vi "GUI_Beampointing2_TRA.vi"() -> ()   [LabVIEW 2013]
uses:
  shared programs/GUI_Template/GUI_master/tcp_new_data_event.ctl
  shared programs/GUI_Template/GUI_master/tcp new data cluster.ctl
  Device Driver/TRAServer/StatusTRA_TypDef.ctl
  Ctrs/beam detection.ctl
  Ctrs/move.ctl
  Ctrs/stats.ctl
  <vilib>/Analysis/NI_AALBase.lvlib
  Device Driver/TRAServer/TRAServer.lvclass
panel:
  in  "Status.Axis 1::2":T1=enum."DISABLE"
  in  "Status.Axis 2::2":T1=enum."DISABLE" caption="Status.Axis 1::2"
  in  "UDP error message":string
  in  "Set Centriod Target":bool
  in  "Tab Control 2":enum32{"CCD Original ", "CCD Detected"}(tab)=enum."CCD Detected"
  out "image::1":T2(plugin-control) caption="StagingM1Far"
  out "Beam":T2(plugin-control)
  in  "Reset History":bool
  out "centriod X":dbl[](graph)=[269.2727355957031, 269.2727355957031, 269.3190002441406]
  out "centriod Y":dbl[](graph)=[287.58294677734375, 287.58294677734375, 287.771484375]
  out "Stats":cluster{timestamp[], dbl[]}[](graph)
  out "move.Stepsize 2":dbl
  out "move.Stepsize":dbl
  in  "Tab Control":enum32{"System", "Detection", "Feedback"}(tab)=enum."Detection"
  in  "Save Stats":bool
  in  "update speed [ms]":i32=200
  in  "img to avg":i32=10
  in  "Save Config":bool
  in  "Load Config":bool
  in  "Cameras":u16(ring)=15 items=["Amp2_surfEast", "Amp2_surfWest", "amp3_surfeast", "amp3_surfwest", "BELLAFrontendCompCam", "Bella_LP_Mode", "Bella_TopviewCCD", "Comp_Final", "EBeam_Profile_BELLA_1", "Flea1_Lanex", "Flea3FW2x2_Lanex", "FLea3Gig_Lanex", "HeatHPDCCD", "HPD_CCD", "LB-FiberCam", "M1-Back-Cam", "M1Cam", "M2Cam", "M3HPD_CCD", "M3HPD_CCD_Near", "M4Cam", "M5Cam", "MagSpecA", "MagSpecB", "MagSpecC", "MagSpecD", "MagSpecE", "MagSpecF", "MagSpecG", "MagSpecH", "MagSpecI", "MagSpecJ", "MagSpecK", "MagSpecL", "P1-SideView", "P2-BlackGuppy", "P2-capspec", "P2-Guppy", "P2-HeatCamPost", "P2-HeatCamPostNear", "P2-HeatCamPreFar", "P2-HeatCamPreFarA", "P2-HeatCamPreNear", "P2-phasics", "P2-phasics151", "P2-ProbeCamPost", "P2-ProbeCamPostNear", "P2-ProbeCamPreNear", "P2-TempCam", "PL1-HexCam", "PL1-phasics151", "PL1-SideSpec", "PL1-TopSpc", "PriyankaCam", "SimCam", "TDBfarfield", "TDBnearfield", "Tel4_Cam", "TPL-Cam-Faraday"]
  in  "wait":u32=200
  in  "beam detection para":T3={"Filter"=1, "Filter Para"={"X Size"=5, "Y Size"=5, "% Tolerance"=1}, "detection method"=4, "smal para"=[{"Measurement Parameter"=35, "Range Lower Value"=0.0, "Range Upper Value"=500.0, "Range"=TRUE, "Measurement Type"=FALSE}], "Remove small Objects"=TRUE, "Restrict to round Objects"=TRUE} {"smal para"."Measurement Parameter" items=["Center of Mass X", "Center of Mass Y", "First Pixel X", "First Pixel Y", "Bounding Rect Left", "Bounding Rect Top", "Bounding Rect Right", "Bounding Rect Bottom", "Max Feret Diameter Start X", "Max Feret Diameter Start Y", "Max Feret Diameter End X", "Max Feret Diameter End Y", "Max Horiz. Segment Length Left", "Max Horiz. Segment Length Right", "Max Horiz. Segment Length Row", "-", "Bounding Rect Width", "Bounding Rect Height", "Bounding Rect Diagonal", "Perimeter", "Convex Hull Perimeter", "Holes' Perimeter", "Max Feret Diameter", "Equivalent Ellipse Major Axis", "Equivalent Ellipse Minor Axis", "Equivalent Ellipse Minor Axis (Feret)", "Equivalent Rect Long Side", "Equivalent Rect Short Side", "Equivalent Rect Diagonal", "Equivalent Rect Short Side (Feret)", "Average Horiz. Segment Length", "Average Vert. Segment Length", "Hydraulic Radius", "Waddel Disk Diameter", "-", "Area", "Holes' Area", "Particle & Holes' Area", "Convex Hull Area", "Image Area", "-", "Number of Holes", "Number of Horiz. Segments", "Number of Vert. Segments", "-", "Orientation", "Max Feret Diameter Orientation", "-", "% Area/Image Area", "% Area/(Particle & Holes' Area)", "Ratio of Equivalent Ellipse Axes", "Ratio of Equivalent Rect Sides", "-", "Elongation Factor", "Compactness Factor", "Heywood Circularity Factor", "Type Factor", "-", "Sum X", "Sum Y", "Sum XX", "Sum XY", "Sum YY", "Sum XXX", "Sum XXY", "Sum XYY", "Sum YYY", "-", "Moment of Inertia XX", "Moment of Inertia XY", "Moment of Inertia YY", "Moment of Inertia XXX", "Moment of Inertia XXY", "Moment of Inertia XYY", "Moment of Inertia YYY", "Norm. Moment of Inertia XX", "Norm. Moment of Inertia XY", "Norm. Moment of Inertia YY", "Norm. Moment of Inertia XXX", "Norm. Moment of Inertia XXY", "Norm. Moment of Inertia XYY", "Norm. Moment of Inertia YYY", "Hu Moment 1", "Hu Moment 2", "Hu Moment 3", "Hu Moment 4", "Hu Moment 5", "Hu Moment 6", "Hu Moment 7"]; "smal para"."Range Lower Value" format="%.2f"; "smal para"."Range Upper Value" format="%.2f"; "detection method" items=["clustering", "entropy", "metric", "moments", "inter-class variance"]; "Filter" items=["No Filter", "Median Filter", "Low Pass Filter"]}
  in  "Move Properties":T5={"Tolerance [%]"=0.1, "Stepsize"=0.0001, "Invert Axis"=TRUE, "Invert Direction X"=FALSE, "Invert Direction Y"=TRUE, "enable feedback"=FALSE, "Set Centriod Target"=FALSE} {"Stepsize" format="%#_6p"}
  out "Y Size":dbl=130.0
  out "X Size":dbl=136.2
  out "Particle Reports (Pixels)":T6(array[cluster])=[{"Area"=12832.0, "Number of Holes"=0.0, "Bounding Rect"={"Left"=200.0, "Top"=223.0, "Right"=335.0, "Bottom"=353.0}, "Center of Mass"={"X"=268.7340243142145, "Y"=287.8902743142145}, "Orientation"=19.894021936277838, "Dimensions"={"Width"=135.0, "Height"=130.0}}] {"Orientation" format="%.2f"; "Dimensions"."Height" format="%.2f"; "Dimensions"."Width" format="%.2f"; "Center of Mass"."Y" format="%.2f"; "Center of Mass"."X" format="%.2f"; "Bounding Rect"."Bottom" format="%.2f"; "Bounding Rect"."Right" format="%.2f"; "Bounding Rect"."Top" format="%.2f"; "Bounding Rect"."Left" format="%.2f"; "Number of Holes" format="%.2f"; "Area" format="%.2f"}
  in  "save cluster":T7={"img to avg"=0, "beam detection para"={"Filter"=0, "Filter Para"={"X Size"=0, "Y Size"=0, "% Tolerance"=0}, "detection method"=0, "smal para"=[], "Remove small Objects"=FALSE, "Restrict to round Objects"=TRUE}, "move"={"Tolerance [%]"=0.1, "Stepsize"=0.0001, "Invert Axis"=TRUE, "Invert Direction X"=FALSE, "Invert Direction Y"=TRUE, "enable feedback"=FALSE, "Set Centriod Target"=FALSE}} {"beam detection para"."smal para"."Measurement Parameter" items=["Center of Mass X", "Center of Mass Y", "First Pixel X", "First Pixel Y", "Bounding Rect Left", "Bounding Rect Top", "Bounding Rect Right", "Bounding Rect Bottom", "Max Feret Diameter Start X", "Max Feret Diameter Start Y", "Max Feret Diameter End X", "Max Feret Diameter End Y", "Max Horiz. Segment Length Left", "Max Horiz. Segment Length Right", "Max Horiz. Segment Length Row", "-", "Bounding Rect Width", "Bounding Rect Height", "Bounding Rect Diagonal", "Perimeter", "Convex Hull Perimeter", "Holes' Perimeter", "Max Feret Diameter", "Equivalent Ellipse Major Axis", "Equivalent Ellipse Minor Axis", "Equivalent Ellipse Minor Axis (Feret)", "Equivalent Rect Long Side", "Equivalent Rect Short Side", "Equivalent Rect Diagonal", "Equivalent Rect Short Side (Feret)", "Average Horiz. Segment Length", "Average Vert. Segment Length", "Hydraulic Radius", "Waddel Disk Diameter", "-", "Area", "Holes' Area", "Particle & Holes' Area", "Convex Hull Area", "Image Area", "-", "Number of Holes", "Number of Horiz. Segments", "Number of Vert. Segments", "-", "Orientation", "Max Feret Diameter Orientation", "-", "% Area/Image Area", "% Area/(Particle & Holes' Area)", "Ratio of Equivalent Ellipse Axes", "Ratio of Equivalent Rect Sides", "-", "Elongation Factor", "Compactness Factor", "Heywood Circularity Factor", "Type Factor", "-", "Sum X", "Sum Y", "Sum XX", "Sum XY", "Sum YY", "Sum XXX", "Sum XXY", "Sum XYY", "Sum YYY", "-", "Moment of Inertia XX", "Moment of Inertia XY", "Moment of Inertia YY", "Moment of Inertia XXX", "Moment of Inertia XXY", "Moment of Inertia XYY", "Moment of Inertia YYY", "Norm. Moment of Inertia XX", "Norm. Moment of Inertia XY", "Norm. Moment of Inertia YY", "Norm. Moment of Inertia XXX", "Norm. Moment of Inertia XXY", "Norm. Moment of Inertia XYY", "Norm. Moment of Inertia YYY", "Hu Moment 1", "Hu Moment 2", "Hu Moment 3", "Hu Moment 4", "Hu Moment 5", "Hu Moment 6", "Hu Moment 7"]; "beam detection para"."smal para"."Range Lower Value" format="%.2f"; "beam detection para"."smal para"."Range Upper Value" format="%.2f"; "beam detection para"."detection method" items=["clustering", "entropy", "metric", "moments", "inter-class variance"]; "beam detection para"."Filter" items=["No Filter", "Median Filter", "Low Pass Filter"]}
  out "move required":bool
  out "moving":bool
  out "Best Rectangle":T8(array[cluster])=[{"Left"=200.0, "Top"=223.0, "Right"=338.0, "Bottom"=353.0}, {"Left"=200.0, "Top"=223.0, "Right"=338.0, "Bottom"=353.0}, {"Left"=205.0, "Top"=224.0, "Right"=338.0, "Bottom"=350.0}, {"Left"=200.0, "Top"=223.0, "Right"=336.0, "Bottom"=355.0}, {"Left"=200.0, "Top"=223.0, "Right"=336.0, "Bottom"=355.0}]
  out "XY Graph":cluster{timestamp[], dbl[]}[](graph)=[{[timestamp(3452404798.8513913 s since 1904-01-01), timestamp(3452404799.6214356 s since 1904-01-01), timestamp(3452404800.2504716 s since 1904-01-01), timestamp(3452404800.877507 s since 1904-01-01), timestamp(3452404801.5115438 s since 1904-01-01), timestamp(3452404802.1385794 s since 1904-01-01), timestamp(3452404802.7796164 s since 1904-01-01), timestamp(3452404803.4086523 s since 1904-01-01), timestamp(3452404804.1166925 s since 1904-01-01), timestamp(3452404804.7627296 s since 1904-01-01), timestamp(3452404805.403766 s since 1904-01-01), timestamp(3452404806.046803 s since 1904-01-01), timestamp(3452404806.8958516 s since 1904-01-01), timestamp(3452404807.531888 s since 1904-01-01), timestamp(3452404808.174925 s since 1904-01-01), timestamp(3452404808.811961 s since 1904-01-01), timestamp(3452404809.4529977 s since 1904-01-01), timestamp(3452404810.0910344 s since 1904-01-01), timestamp(3452404810.732071 s since 1904-01-01), timestamp(3452404811.373108 s since 1904-01-01)], [-3.53924560546875, -4.652754657642788, -5.44743290091867, -5.300940785876151, -4.715238659785825, -6.004101011596333, -4.752166041728003, -5.050226506875958, -4.109178710453193, -4.665509033203136, -5.175085449218727, -5.028265380859352, -4.379766845703102, -4.631829833984398, -4.844409179687489, -4.304394531250011, -4.530322265624989, -4.936749267578136, -4.763983154296852, -4.448400878906227]}, {[timestamp(3452404798.8513913 s since 1904-01-01), timestamp(3452404799.6214356 s since 1904-01-01), timestamp(3452404800.2504716 s since 1904-01-01), timestamp(3452404800.877507 s since 1904-01-01), timestamp(3452404801.5115438 s since 1904-01-01), timestamp(3452404802.1385794 s since 1904-01-01), timestamp(3452404802.7796164 s since 1904-01-01), timestamp(3452404803.4086523 s since 1904-01-01), timestamp(3452404804.1166925 s since 1904-01-01), timestamp(3452404804.7627296 s since 1904-01-01), timestamp(3452404805.403766 s since 1904-01-01), timestamp(3452404806.046803 s since 1904-01-01), timestamp(3452404806.8958516 s since 1904-01-01), timestamp(3452404807.531888 s since 1904-01-01), timestamp(3452404808.174925 s since 1904-01-01), timestamp(3452404808.811961 s since 1904-01-01), timestamp(3452404809.4529977 s since 1904-01-01), timestamp(3452404810.0910344 s since 1904-01-01), timestamp(3452404810.732071 s since 1904-01-01), timestamp(3452404811.373108 s since 1904-01-01)], [1.230804443359375, -0.3328436558336989, 0.6609996983648898, -0.3690822614664171, 0.27569034847687135, -0.11031780080207909, -0.31644478020683664, 0.5764054032015906, 0.6783385802021371, 0.532257080078125, 0.9677673339843977, 0.27269287109373863, 0.38755493164063637, 0.46185302734375, 0.137542724609375, 0.073089599609375, 0.6028076171875227, 0.7097961425781136, 1.0255981445312727, 0.9409057617187386]}]
  out "Y offset":dbl=0.9409057617187386
  out "X offset":dbl=-4.448400878906227
  in  "Target.X::1":dbl=265.0 min=0.0 max=2000.0 format="%#_6f"
  in  "Target.Y::1":dbl=288.0 min=0.0 max=2000.0 format="%#_6f"
  out "mean Y":dbl=287.05909423828126 format="%0.2f"
  out "mean X":dbl=269.4484008789062 format="%0.2f"
  out "beam detected":bool=TRUE
  out "Status.Axis 4::2":T1=enum."DISABLE" caption="Status.Axis 1::2"
  in  "Status.Axis 3::2":T1=enum."DISABLE" caption="Status.Axis 1::2"
  in  "Position.Axis 1::2":dbl=1.39334 caption="TREX M20 X" min=0.0 max=6.0 format="%#_6f"
  in  "Position.Axis 2::2":dbl=4.66198 caption="TREX M20 Y" min=0.0 max=7.0 format="%#_6f"
  in  "GUIdevice 2":string="TREX TRA1"
  out "error out":errorcluster
  in  "insert tag":bool=TRUE
  in  "stop":bool=TRUE
  in  "GUIdevice 1":string="StagingM1Near"
  out "tcp data event":T9
  out "error IO 2":errorcluster
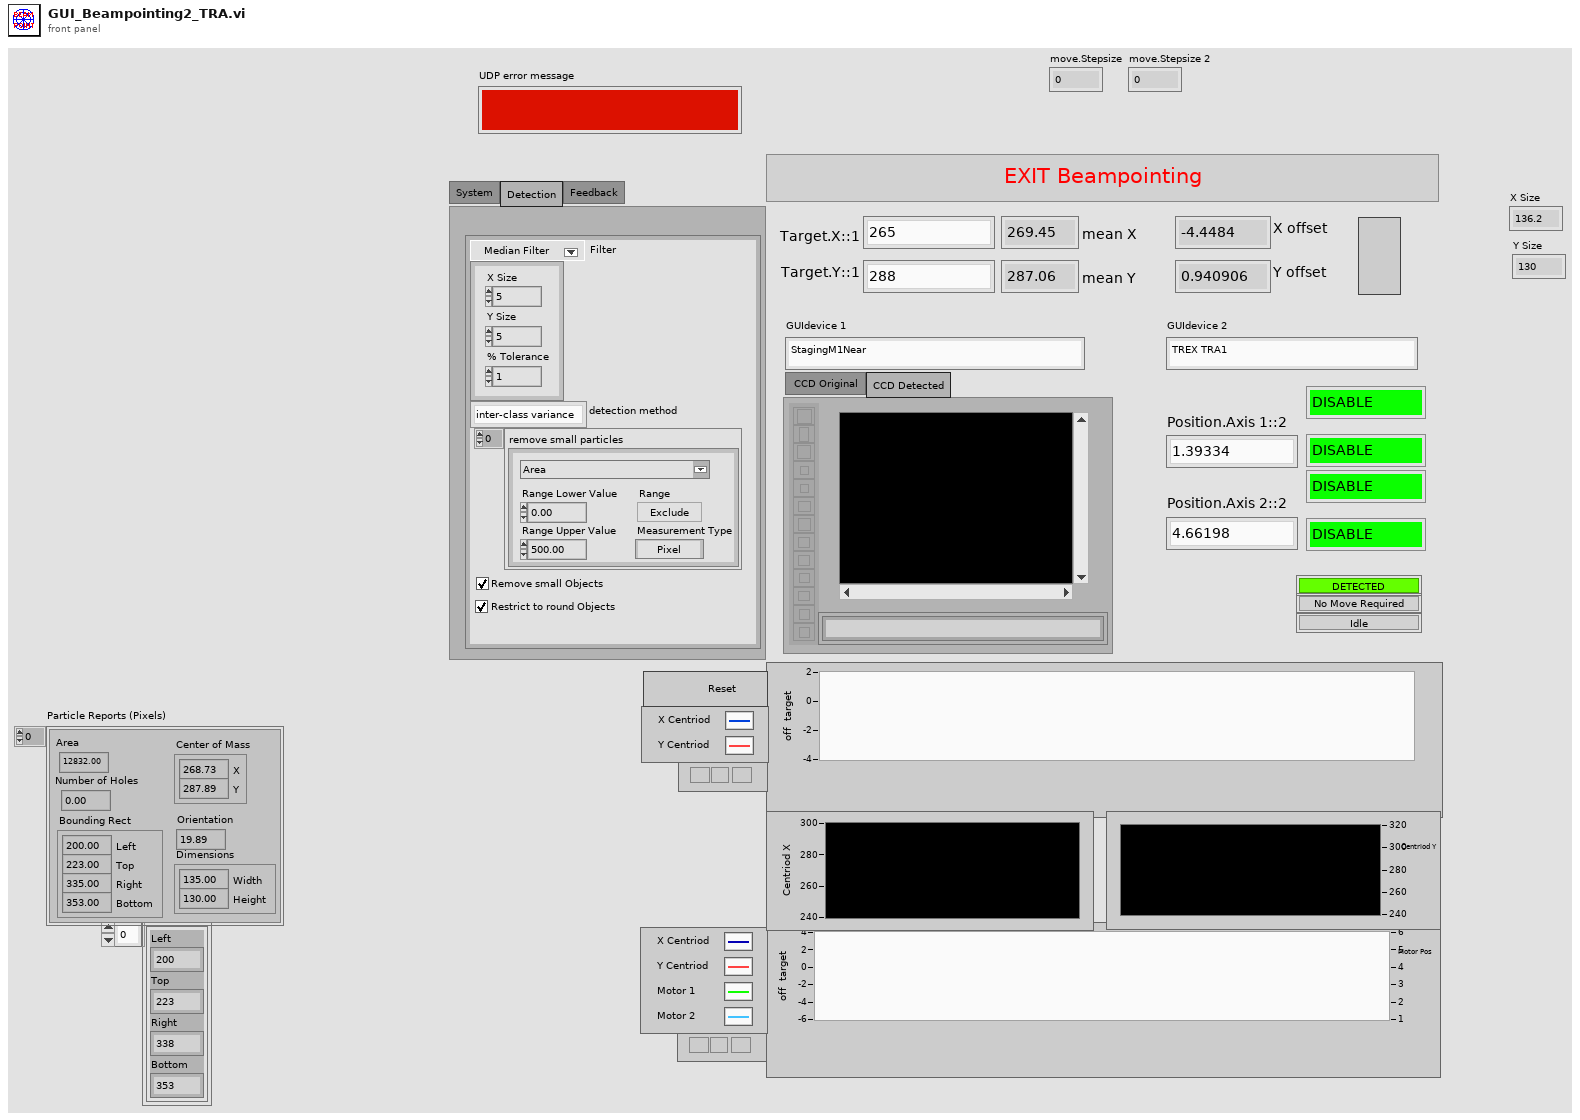
[diagram p1: front panel]
types:
  T1 = typedef "TRAServer.lvclass/StatusTRA_TypDef.ctl" = enum16{"NOT REFERENCED", "CONFIGURATION", "HOMING", "MOVING", "READY", "DISABLE", "JOGGING"}
  T2 = typedef "IMAQ Image.ctl" = refnum<image>
  T3 = typedef "beam detection.ctl" = cluster{"Filter":u16, "Filter Para":cluster{"X Size":i32, "Y Size":i32, "% Tolerance":i32}, "detection method":i32, "smal para":cluster{"Measurement Parameter":T4, "Range Lower Value":dbl, "Range Upper Value":dbl, "Range":bool, "Measurement Type":bool}[], "Remove small Objects":bool, "Restrict to round Objects":bool}
  T4 = typedef "Particle Parameters" = i32
  T5 = typedef "move.ctl" = cluster{"Tolerance [%]":dbl, "Stepsize":dbl, "Invert Axis":bool, "Invert Direction X":bool, "Invert Direction Y":bool, "enable feedback":bool, "Set Centriod Target":bool}
  T6 = cluster{"Area":dbl, "Number of Holes":dbl, "Bounding Rect":cluster{"Left":dbl, "Top":dbl, "Right":dbl, "Bottom":dbl}, "Center of Mass":cluster{"X":dbl, "Y":dbl}, "Orientation":dbl, "Dimensions":cluster{"Width":dbl, "Height":dbl}}[]
  T7 = cluster{"img to avg":i32, "beam detection para":T3, "move":T5}
  T8 = cluster{"Left":dbl, "Top":dbl, "Right":dbl, "Bottom":dbl}[]
  T9 = typedef "tcp_new_data_event.ctl" = refnum<user-event>
  T10 = typedef "tcp new data cluster.ctl" = cluster{"EventEnum":enum16{"new data", "connection status update"}, "Device name":string}
  T11 = typedef "Image Type" = u32
  T12 = cluster{"Left":i32, "Top":i32, "Right":i32, "Bottom":i32}
  T13 = enum32{"invalid app kind", "Development System", "Run Time System", "Student Edition", "Embedded LabVIEW", "Evaluation", "Custom"}
  T14 = enum32{"Invalid", "Standard", "Closed", "Hidden", "Minimized", "Maximized"}
  T15 = enum16{"open", "replace", "create", "open or create", "replace or create", "replace or create with confirmation"}
  T16 = typedef "stats.ctl" = cluster{"Stat Centriod X":dbl[], "Stat Centriod Y":dbl[], "TRA Position X":dbl[], "TRA PositionY":dbl[], "Time":timestamp[]}
  T17 = cluster{"Core":cluster{"Current VI Reference":refnum<vi>, "Close Panel on Exit?":bool}, "beam detection para":T3, "Centriod X":dbl[], "Centriod Y":dbl[], "Best Rectangle":cluster{"Left":dbl, "Top":dbl, "Right":dbl, "Bottom":dbl}[], "PArticle Report":cluster{"Area":dbl, "Number of Holes":dbl, "Bounding Rect":cluster{"Left":dbl, "Top":dbl, "Right":dbl, "Bottom":dbl}, "Center of Mass":cluster{"X":dbl, "Y":dbl}, "Orientation":dbl, "Dimensions":cluster{"Width":dbl, "Height":dbl}}[], "Mean Centriod X":dbl[], "Mean Centriod Y":dbl[], "Time":timestamp[], "beam detected":bool, "offsets":cluster{"X offset":dbl, "Y offset":dbl}, "move":T5, "moving":bool, "Stats":T16, "set centriod target":bool}
  T18 = cluster{"Left":dbl, "Top":dbl, "Right":dbl, "Bottom":dbl}
  T19 = cluster{"Current VI Reference":refnum<vi>, "Close Panel on Exit?":bool}
  T20 = cluster{"Time":timestamp[], "Stat Centriod X":dbl[]}
  T21 = cluster{"Time":timestamp[], "Stat Centriod Y":dbl[]}
  T22 = cluster{"Time":timestamp[], "TRA Position X":dbl[]}
  T23 = cluster{"Time":timestamp[], "TRA PositionY":dbl[]}
  T24 = cluster{"Time":timestamp[], "TRA PositionY":dbl[]}[]
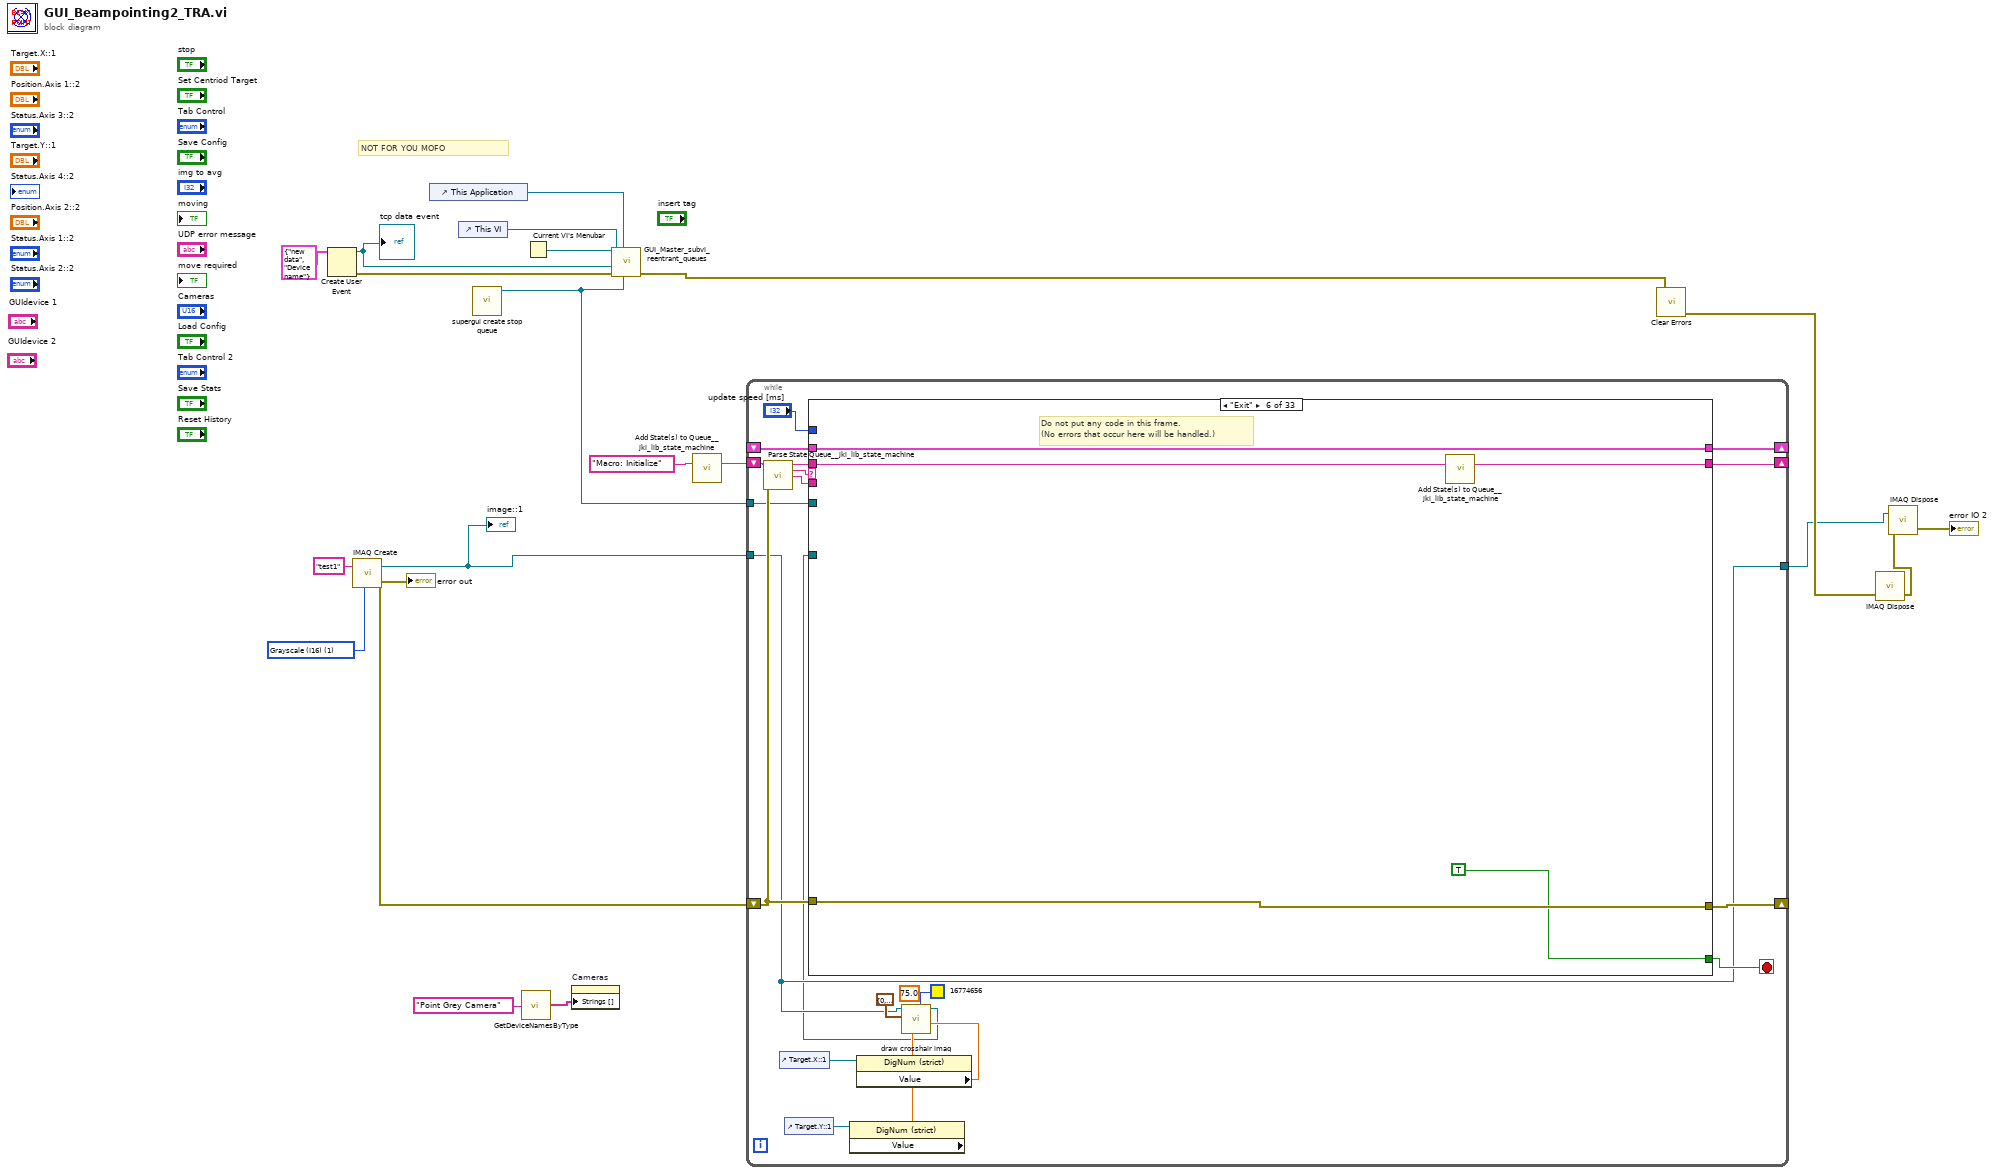
[diagram p0: block diagram]
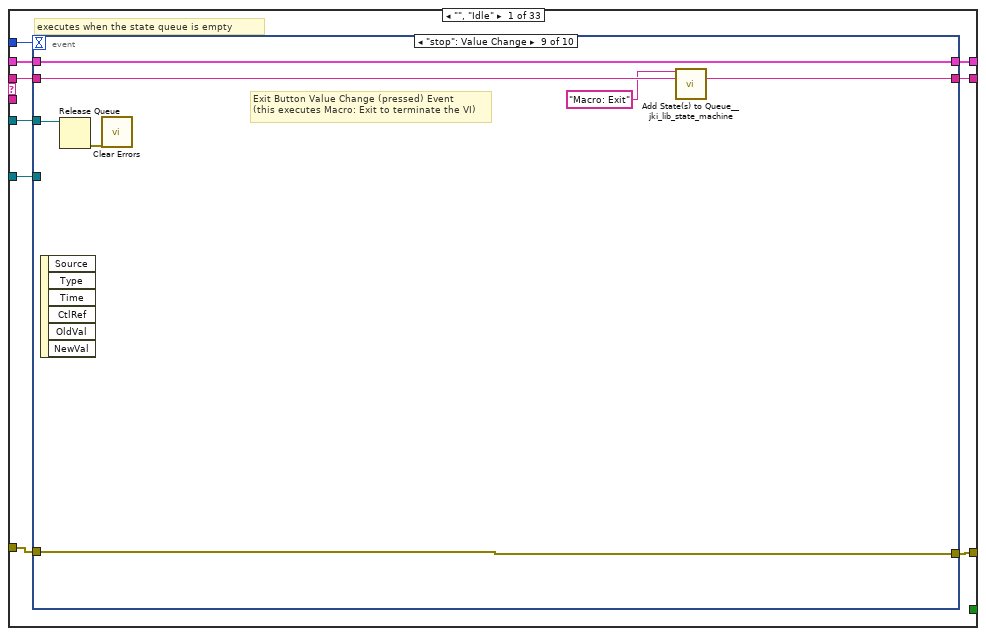
[diagram p2: hidden frame]
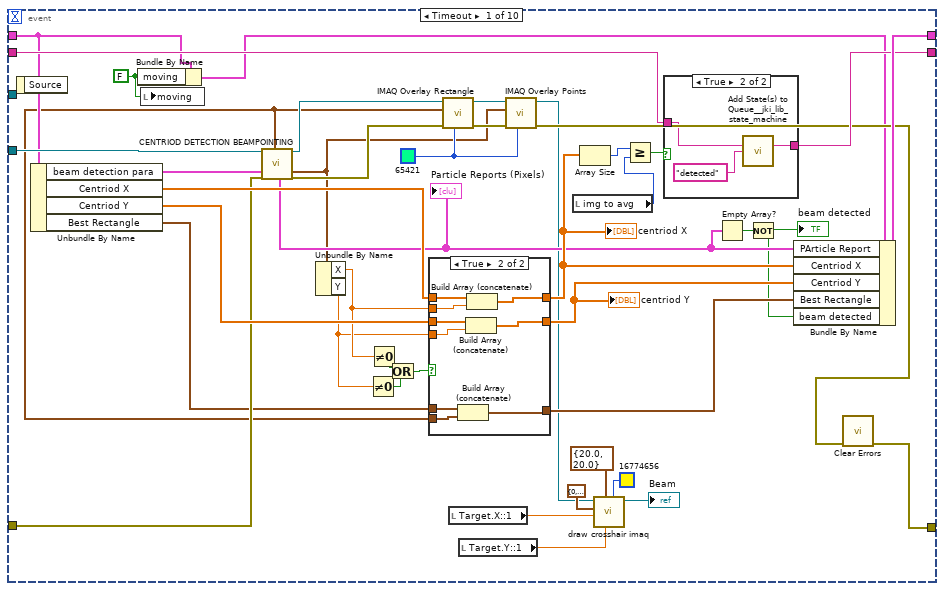
[diagram p3: hidden frame]
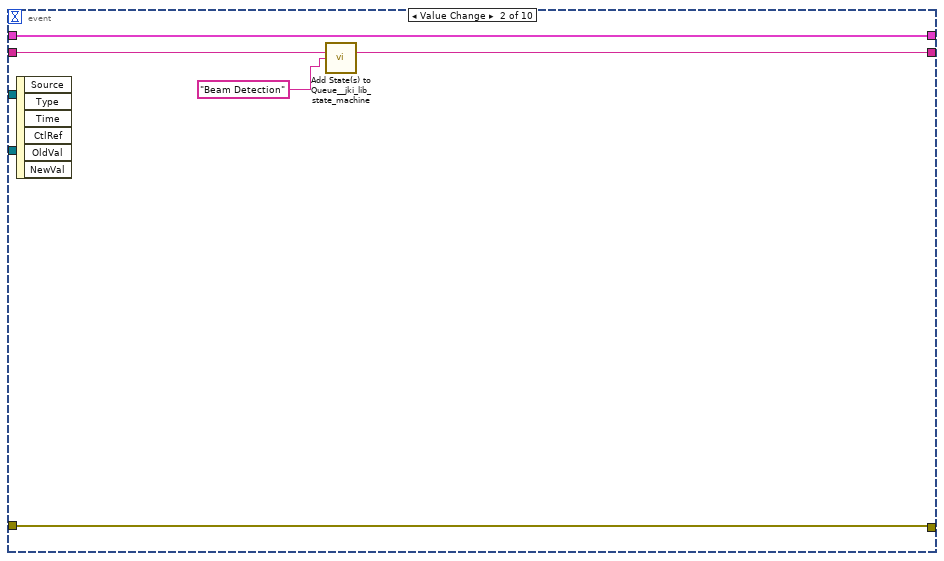
[diagram p6: hidden frame]
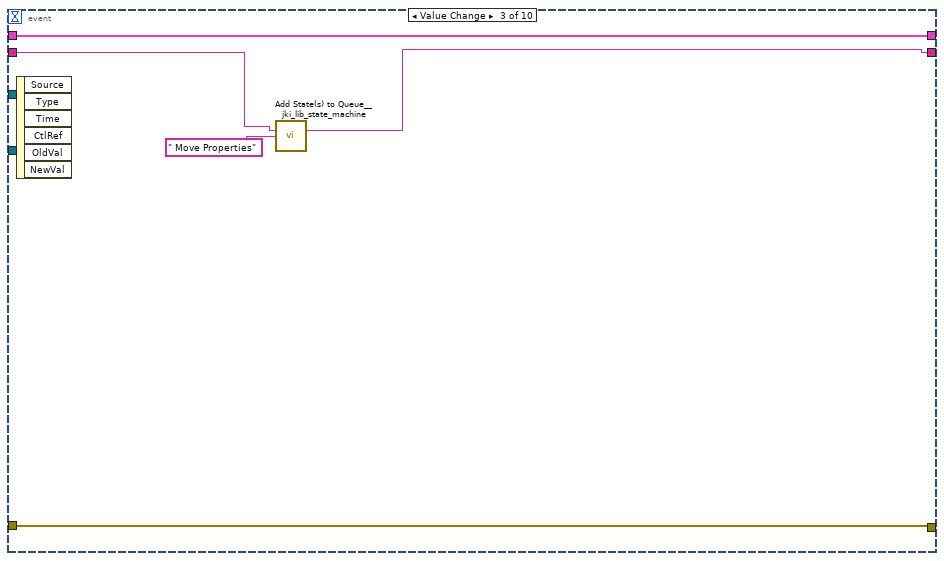
[diagram p7: hidden frame]
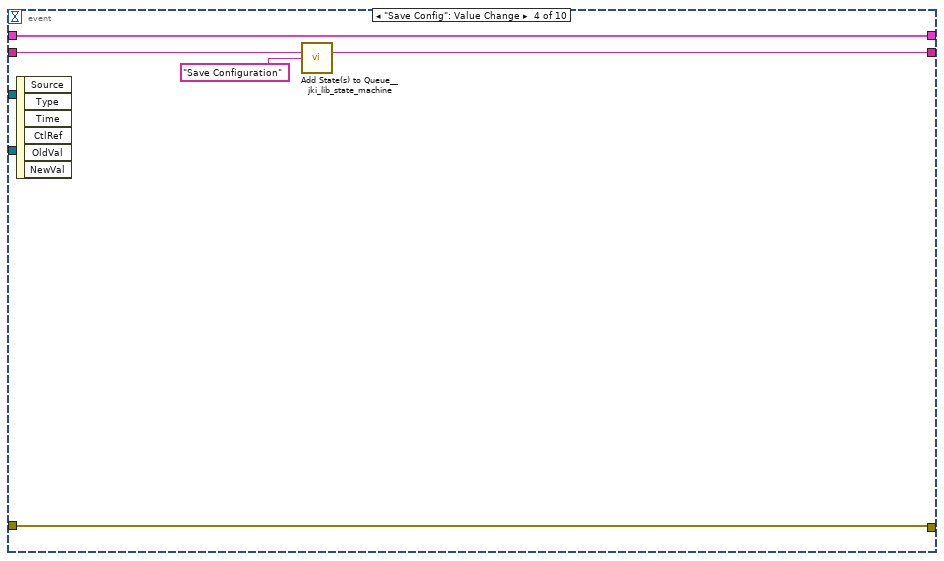
[diagram p8: hidden frame]
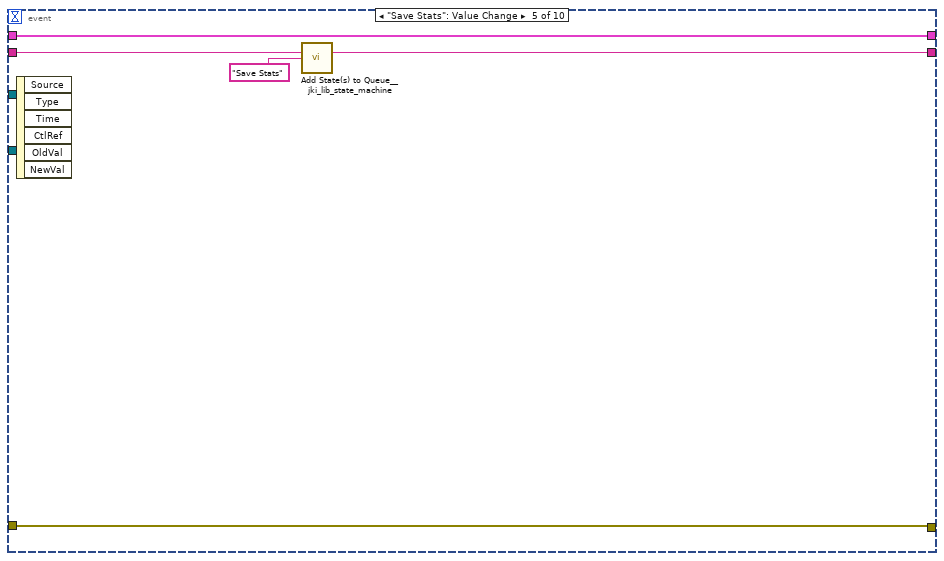
[diagram p9: hidden frame]
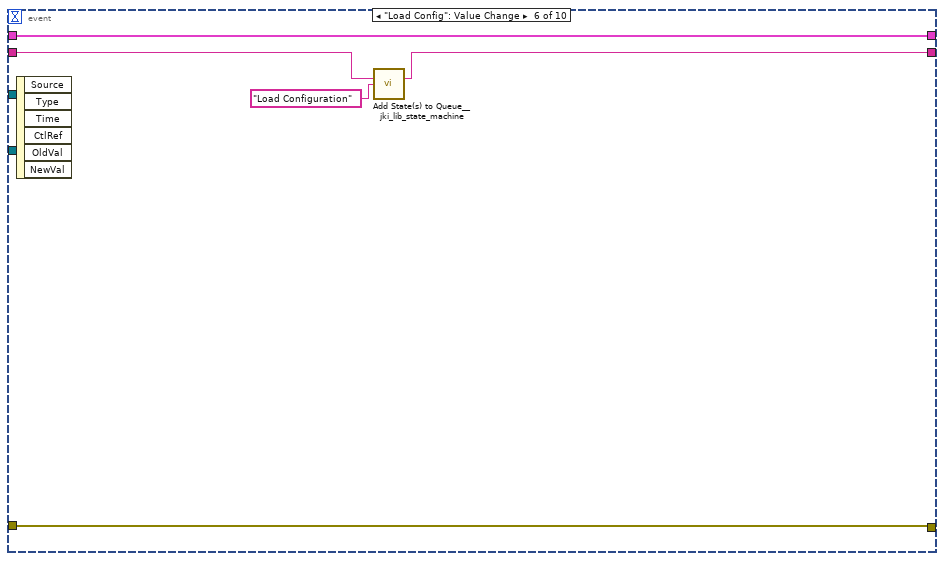
[diagram p10: hidden frame]
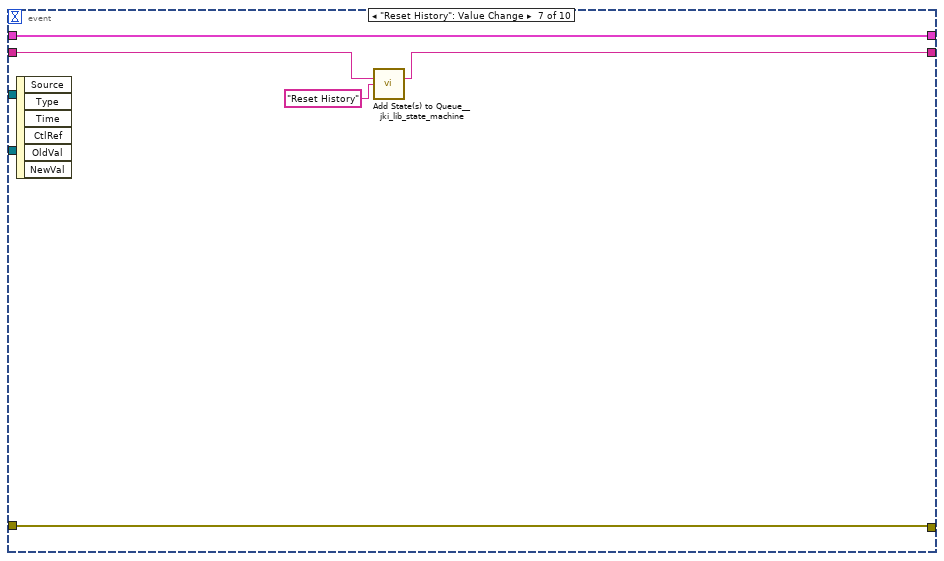
[diagram p11: hidden frame]
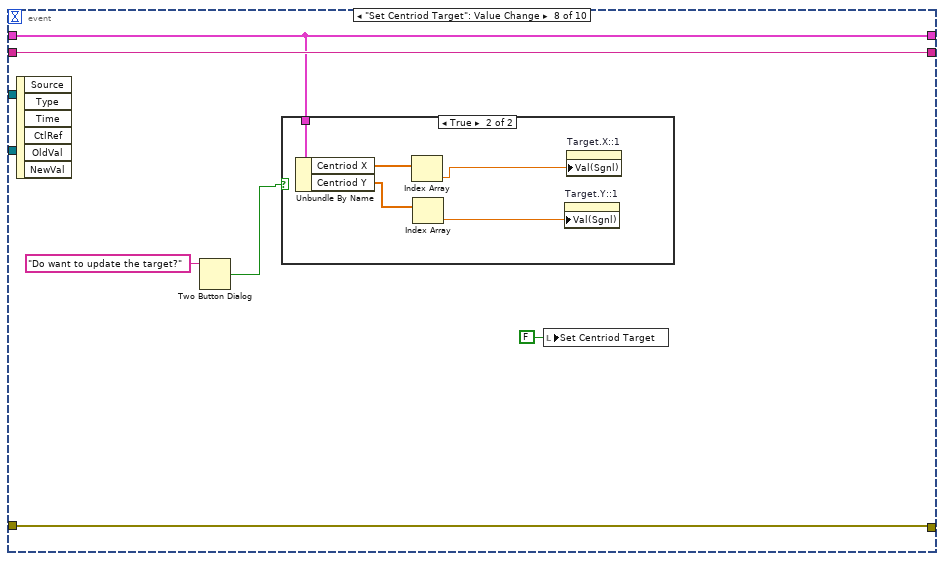
[diagram p12: hidden frame]
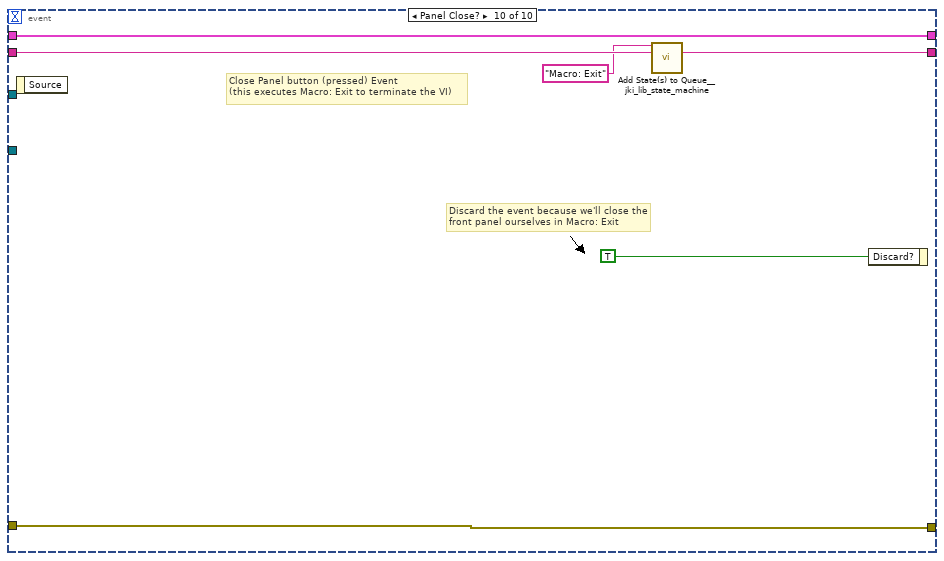
[diagram p14: hidden frame]
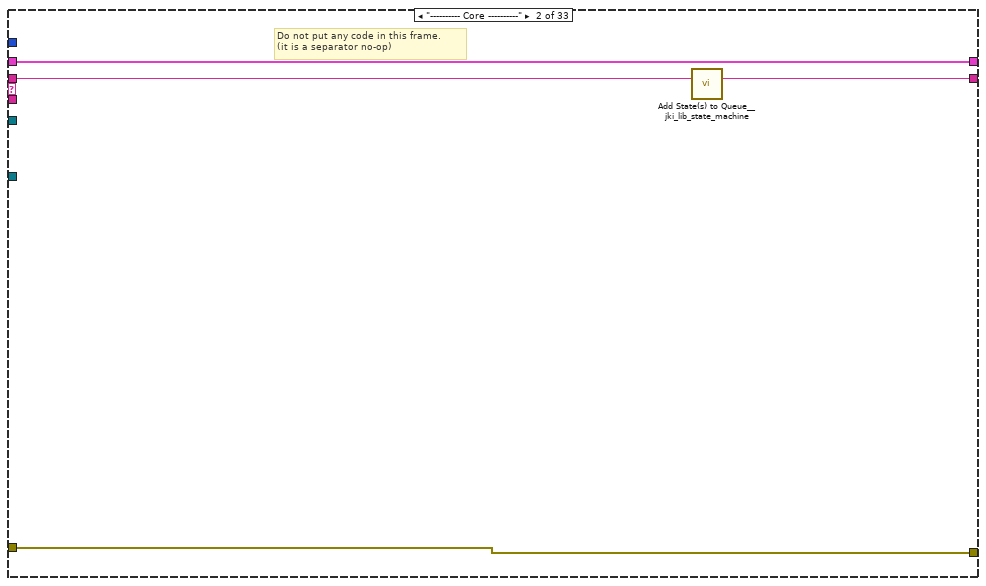
[diagram p15: hidden frame]
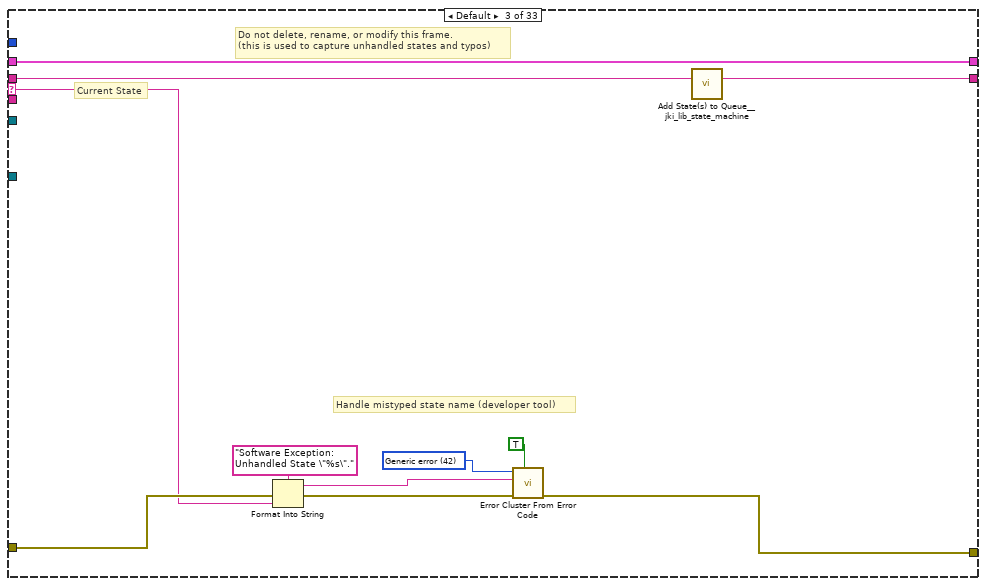
[diagram p16: hidden frame]
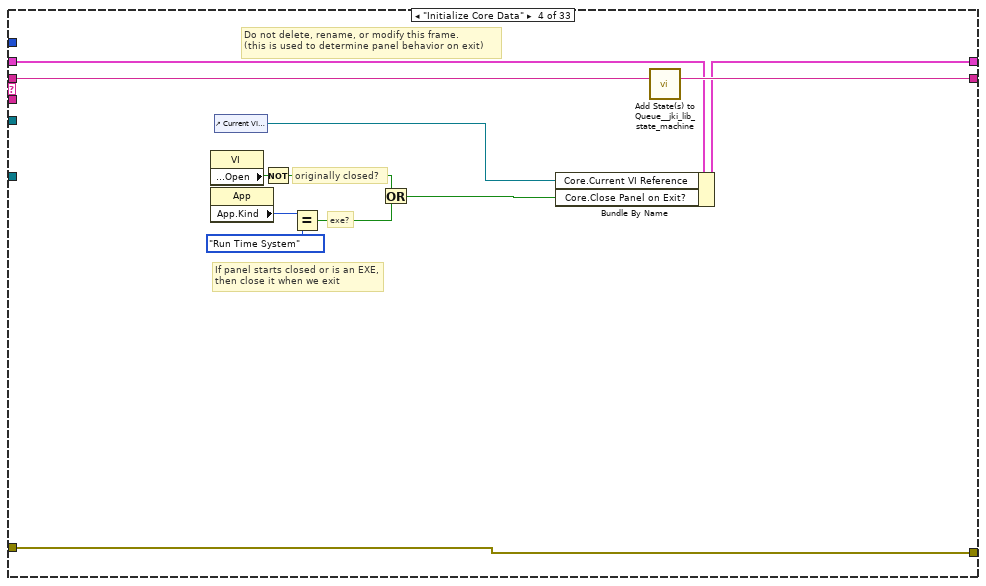
[diagram p17: hidden frame]
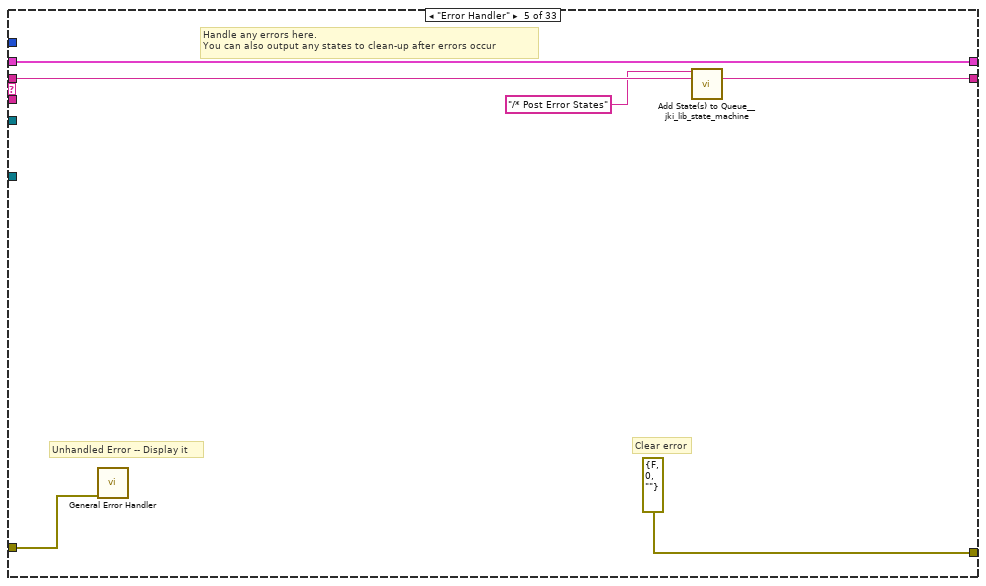
[diagram p18: hidden frame]
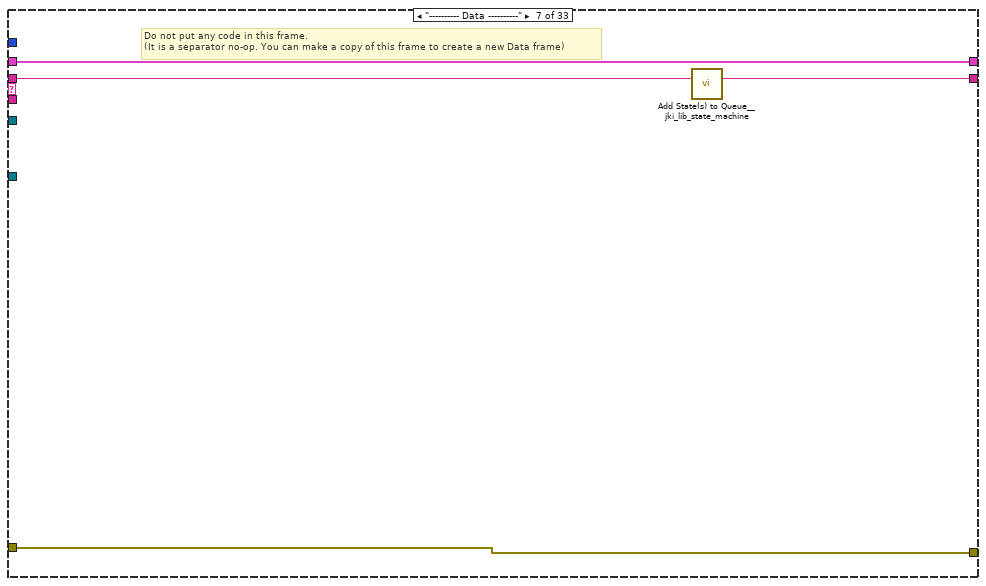
[diagram p19: hidden frame]
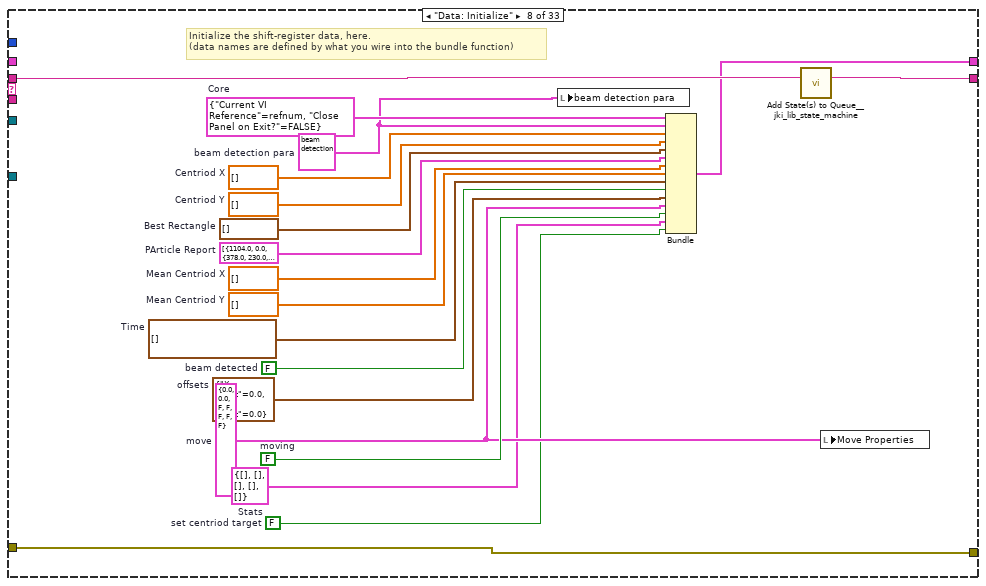
[diagram p20: hidden frame]
diagram:
  w19 = T11 1 items=["Grayscale (U8)", "Grayscale (I16)", "Grayscale (SGL)", "Complex (CSG)", "RGB (U32)", "HSL (U32)", "RGB (U64)", "Grayscale (U16)"] ("Image Type")
  # "NOT FOR YOU MOFO"
  n1 = Create User Event(user event datatype=T10 {"EventEnum"=enum."new data", "Device name"="Device name"} ("New Event")) -> (user event=w5:refnum<user-event>, error out=w7:errorcluster)  [unwired: 1 in]
  "tcp data event" <- w5
  n2 = call "IMAQ Create"("Image Name"="test1", "Image Type"=w19) -> ("New Image"=w4:T2, "error out"=w12:errorcluster)  [unwired: 3 in]
  "error out" <- w12
  "image::1" <- w4
  n3 = control-ref of="This Application"() -> (w6:refnum<vi>)
  n4 = control-ref of="This VI"() -> (w10:refnum<vi>)
  n5 = call "supergui create stop queue.vi"() -> ("STOP Queue out"=w1:refnum<queue>)  [unwired: 11 in]
  n6 = call "GetDeviceNamesByType.vi"("Device Type"="Point Grey Camera") -> ("Array"=w2:string[])
  n7 = Current VI's Menubar() -> (w9:refnum<k9>)
  n8 = property on="Cameras" class="Ring (strict)"("Strings []"=w2) -> ()  [unwired: 2 in, 2 out]
  n9 = call "GUI_Master_subvi_reentrant_queues.vi"("STOP Queue in"=w1, "This Application"=w6, "error in (no error)"=w7, "tcp data event"=w5, "Caller menu reference"=w9, "Caller VI ref"=w10) -> ("error out"=w18:errorcluster)  [unwired: 5 in]
  n10 = call <vilib>:"Add State(s) to Queue__jki_lib_state_machine.vi"("State(s) in (\"\")"="Macro: Initialize") -> ("States Out"=w14:string)  [unwired: 14 in]
  n11 = while "JKI - String-Based Queued State Machine (Basic) v1.0" {
    shift-right: [w34] -> _
    shift-left: _ -> [w33]
    shift-right: [w36] -> _
    shift-left: w12 -> [w31]
    shift-right: [w35] -> _
    shift-left: w14 -> [w37]
    tunnel: w4 -> [w23]
    tunnel: [w23] -> w11
    tunnel: w1 -> [w21]
    stop <- w30 stop-if-true
    (unwired) 75.0 ("size")
    n12 = call <vilib>:"Parse State Queue__jki_lib_state_machine.vi"("State Queue"=w37, "Error In (no error)"=w31) -> ("Remaining States"=w39:string, "Current State"=w40:string, "Arguments"=w38:string)  [unwired: 11 in]
    n13 = control-ref of="Target.X::1"() -> (w26:refnum<vi>)
    n14 = control-ref of="Target.Y::1"() -> (w27:refnum<vi>)
    n15 = property class="DigNum (strict)"(reference=w27) -> ("Value"=w29:dbl)  [unwired: 1 in, 2 out]
    n16 = property class="DigNum (strict)"(reference=w26) -> ("Value"=w28:dbl)  [unwired: 1 in, 2 out]
    n17 = call "draw crosshair imaq.vi"("Color"=u32 16774656, "Target.Y"=w29, "Target.X"=w28, "Bounding Rectangle"=T12 {"Left"=0, "Top"=0, "Right"=0, "Bottom"=0}, "image in"=w23) -> ("image out"=w22:T2)  [unwired: 5 in, 1 out]
    n18 = case shown="\"Exit\"" w40 {
      selector: w40 -> [_ _ w166 _ _ _ _ _ _ _ _ _ _ _ _ _ _ _ _ _ _ _ _ _ _ _ _ _ _ _ _ _ _]
      tunnel: w39 -> [w49 w165 w170 w188 w194 w199 w203 w222 w228 w232 w236 w242 w253 w279 w284 w294 w298 w304 w310 w325 w337 w353 w360 w364 w391 w396 w434 w447 w492 w532 w548 w590 w594]
      tunnel: w38 -> [_ _ _ _ _ _ _ _ _ _ _ w237 w247 _ _ _ _ _ _ _ _ _ _ _ _ _ _ _ _ _ _ _ _]
      tunnel: w33 -> [w47 w162 w168 w179 w191 w197 w200 _ w224 w229 w234 w240 w249 w276 w281 w291 w295 w300 w306 w321 w333 w344 w356 w361 w371 w398 w431 w437 w483 w529 w545 w582 w591]
      tunnel: [w46 w163 w172 w185 errorcluster {"status"=FALSE, "code"=0, "source"=""} ("error out") w196 w201 w219 w225 w230 w233 w238 w250 w277 w282 w292 w296 w302 w308 w312 w328 w341 w358 w362 w389 w417 w432 w445 w490 w530 w546 w588 w592] -> w36
      tunnel: w31 -> [w45 w163 w171 w185 w190 w196 w201 w219 w226 w230 w233 w239 w251 w277 w282 w292 w296 w302 w308 w313 w329 w342 w358 w362 w389 w417 w432 w445 w490 w530 w546 w588 w592]
      tunnel: [w48 w164 w169 w187 w193 w198 w202 w221 w227 w231 w235 w241 w252 w278 w283 w293 w297 w303 w309 w324 w336 w352 w359 w363 w390 w404 w433 w446 w491 w531 w547 w589 w593] -> w35
      tunnel: [_ _ _ _ _ TRUE _ _ _ _ _ _ _ _ _ _ _ _ _ _ _ _ _ _ _ _ _ _ _ _ _ _ _] -> w30
      tunnel: [w44 w162 w168 w186 w191 w197 w200 w220 w224 w229 w234 w240 w249 w276 w281 w291 w295 w299 w305 w321 w333 w343 w355 w361 w370 w402 w431 w439 w482 w527 w544 w571 w591] -> w34
      tunnel: "update speed [ms]" -> [w43 _ _ _ _ _ _ _ _ _ _ _ _ _ _ _ _ _ _ _ _ _ _ _ _ _ _ _ _ _ _ _ _]
      tunnel: w22 -> [w42 _ _ _ _ _ _ _ _ _ _ _ _ _ _ _ _ _ _ _ _ _ _ _ _ _ _ _ _ _ _ _ _]
      tunnel: w21 -> [w41 _ _ _ _ _ _ _ _ _ _ _ _ _ _ _ _ _ _ _ _ _ _ _ _ _ _ _ _ _ _ _ _]
      frame "", "Idle" {
        # "executes when the state queue is empty"
        n19 = event shown="[8] \"stop\": Value Change" {
          selector: _ -> [_ _ _ _ _ _ _ _ _ _]
          dyn-events: _ -> [_ _ _ _ _ _ _ _ _ _]
          timeout: w43 -> [_ _ _ _ _ _ _ _ _ _]
          tunnel: w49 -> [w71 w111 w116 w121 w126 w130 w135 w142 w155 w161]
          tunnel: [w70 w110 w114 w119 w124 w129 w134 w142 w154 w160] -> w48
          tunnel: w47 -> [w61 w112 w117 w122 w127 w132 w137 w141 w152 w158]
          tunnel: [w67 w109 w113 w118 w123 w131 w136 w143 w153 w159] -> w46
          tunnel: w45 -> [w86 w109 w113 w118 w123 w131 w136 w143 w153 w159]
          tunnel: [w89 w112 w117 w122 w127 w132 w137 w141 w152 w158] -> w44
          tunnel: w42 -> [w90 _ _ _ _ _ _ _ _ _]
          tunnel: w41 -> [_ _ _ _ _ _ _ _ w150 _]
          event Timeout {
            w59 = FALSE ("moving")
            w78 = u32 65421 ("Color")
            n20 = event-data() -> ()  [unwired: 1 in, 1 out]
            n21 = Unbundle By Name(w61) -> ("beam detection para"=w91:T3, "Centriod X"=w88:dbl[], "Centriod Y"=w87:dbl[], "Best Rectangle"=w80:T8)
            n22 = Bundle By Name(cluster=w61, "moving"=w59) -> (w60:T17)
            n23 = local write "moving"(w59) -> ()
            n24 = call "CENTRIOD DETECTION BEAMPOINTING.vi"("Refnum in"=w90, "beam detection para"=w91, "error in (no error)"=w86) -> ("Bounding Rect"=w51:T18, "Particle Reports (Pixels)"=w64:T6, "Refnum out"=w75:T2, "Centriod"=w52:cluster{"X":dbl, "Y":dbl}, "error out"=w69:errorcluster)  [unwired: 10 in, 2 out]
            "Particle Reports (Pixels)" <- w64
            n25 = Unbundle By Name(w52) -> ("X"=w83:dbl, "Y"=w82:dbl)
            n26 = Not Equal To 0?(x=w82) -> (x != 0?=w85:bool)
            n27 = Not Equal To 0?(x=w83) -> (x != 0?=w84:bool)
            n28 = Or(x=w84, y=w85) -> (x .or. y?=w81:bool)
            n29 = case shown="True" w81 {
              tunnel: w88 -> [w98 w107]
              tunnel: w87 -> [w97 w106]
              tunnel: [w98 w105] -> w73
              tunnel: [w97 w104] -> w74
              tunnel: w83 -> [_ w103]
              tunnel: w82 -> [_ w102]
              tunnel: w80 -> [w96 w101]
              tunnel: w51 -> [_ w100]
              tunnel: [w96 w99] -> w79
              frame False {
              }
              frame True {
                n30 = Build Array (concatenate)(w101, w100) -> (w99:T8)
                n31 = Build Array (concatenate)(w106, w102) -> (w104:dbl[])
                n32 = Build Array (concatenate)(w107, w103) -> (w105:dbl[])
              }
            }
            "centriod X" <- w73
            "centriod Y" <- w74
            n33 = call "IMAQ Overlay Rectangle"("Color"=w78, "error in (no error)"=w69, "Rectangle"=w51, "Image"=w75) -> ("error out"=w76:errorcluster, "Image Out"=w77:T2)  [unwired: 6 in]
            n34 = local read "Target.X::1"() -> (w54:dbl)
            n35 = local read "Target.Y::1"() -> (w53:dbl)
            n36 = call "IMAQ Overlay Points"("Color"=w78, "error in (no error)"=w76, "Point"=w52, "Image"=w77) -> ("error out"=w68:errorcluster, "Image Out"=w56:T2)  [unwired: 6 in]
            n37 = local read "img to avg"() -> (w65:i32)
            n38 = Array Size(array=w73) -> (size(s)=w66:i32)
            n39 = call "draw crosshair imaq.vi"("Color"=u32 16774656, "Target.Y"=w53, "size"=cluster{"xhair size":dbl, "xhair size 2":dbl} {"xhair size"=20.0, "xhair size 2"=20.0}, "Target.X"=w54, "Bounding Rectangle"=T12 {"Left"=0, "Top"=0, "Right"=0, "Bottom"=0}, "image in"=w56) -> ("image out"=→"Beam":T2)  [unwired: 4 in, 1 out]
            n40 = Greater Or Equal?(x=w66, y=w65) -> (x >= y?=w72:bool)
            n41 = case shown="True" w72 {
              tunnel: w71 -> [w92 w95]
              tunnel: [w92 w94] -> w70
              frame False {
              }
              frame True {
                n42 = call <vilib>:"Add State(s) to Queue__jki_lib_state_machine.vi"("State(s) in (\"\")"=w95, "State(s) at Back (\"\")"="detected" ("State(s) in Front (\"\")")) -> ("States Out"=w94:string)  [unwired: 13 in]
              }
            }
            n43 = Empty Array?(array=w64) -> (empty?=w63:bool)
            n44 = Not(x=w63) -> (.not. x?=w62:bool)
            "beam detected" <- w62
            n45 = Bundle By Name(cluster=w60, "PArticle Report"=w64, "Centriod X"=w73, "Centriod Y"=w74, "Best Rectangle"=w79, "beam detected"=w62) -> (w89:T17)
            n46 = call <vilib>:"Clear Errors.vi"("error in (no error)"=w68) -> ("error out"=w67:errorcluster)  [unwired: 6 in]
          }
          event Value Change {
            n47 = event-data() -> ()  [unwired: 1 in, 6 out]
            n48 = call <vilib>:"Add State(s) to Queue__jki_lib_state_machine.vi"("State(s) in (\"\")"=w111, "State(s) at Back (\"\")"="Beam Detection" ("State(s) at Back (\"\")")) -> ("States Out"=w110:string)  [unwired: 13 in]
          }
          event Value Change {
            n49 = event-data() -> ()  [unwired: 1 in, 6 out]
            n50 = call <vilib>:"Add State(s) to Queue__jki_lib_state_machine.vi"("State(s) in (\"\")"=w116, "State(s) at Back (\"\")"=" Move Properties" ("State(s) at Back (\"\")")) -> ("States Out"=w114:string)  [unwired: 13 in]
          }
          event "Save Config": Value Change {
            n51 = event-data() -> ()  [unwired: 1 in, 6 out]
            n52 = call <vilib>:"Add State(s) to Queue__jki_lib_state_machine.vi"("State(s) in (\"\")"=w121, "State(s) at Back (\"\")"="Save Configuration" ("State(s) in Front (\"\")")) -> ("States Out"=w119:string)  [unwired: 13 in]
          }
          event "Save Stats": Value Change {
            n53 = event-data() -> ()  [unwired: 1 in, 6 out]
            n54 = call <vilib>:"Add State(s) to Queue__jki_lib_state_machine.vi"("State(s) in (\"\")"=w126, "State(s) at Back (\"\")"="Save Stats" ("State(s) in Front (\"\")")) -> ("States Out"=w124:string)  [unwired: 13 in]
          }
          event "Load Config": Value Change {
            n55 = event-data() -> ()  [unwired: 1 in, 6 out]
            n56 = call <vilib>:"Add State(s) to Queue__jki_lib_state_machine.vi"("State(s) in (\"\")"=w130, "State(s) at Back (\"\")"="Load Configuration" ("State(s) in Front (\"\")")) -> ("States Out"=w129:string)  [unwired: 13 in]
          }
          event "Reset History": Value Change {
            n57 = event-data() -> ()  [unwired: 1 in, 6 out]
            n58 = call <vilib>:"Add State(s) to Queue__jki_lib_state_machine.vi"("State(s) in (\"\")"=w135, "State(s) at Back (\"\")"="Reset History" ("State(s) in Front (\"\")")) -> ("States Out"=w134:string)  [unwired: 13 in]
          }
          event "Set Centriod Target": Value Change {
            n59 = event-data() -> ()  [unwired: 1 in, 6 out]
            n60 = Two Button Dialog(message="Do want to update the target?") -> (T button?=w138:bool)  [unwired: 2 in]
            n61 = case shown="True" w138 {
              tunnel: w141 -> [_ w148]
              frame False {
              }
              frame True {
                n62 = Unbundle By Name(w148) -> ("Centriod X"=w147:dbl[], "Centriod Y"=w145:dbl[])
                n63 = Index Array(array=w147) -> (element=w146:dbl)  [unwired: 1 in]
                n64 = Index Array(array=w145) -> (element=w144:dbl)  [unwired: 1 in]
                n65 = property on="Target.Y::1" class="DigNum (strict)"("Val(Sgnl)"=w144) -> ()  [unwired: 2 in, 2 out]
                n66 = property on="Target.X::1" class="DigNum (strict)"("Val(Sgnl)"=w146) -> ()  [unwired: 2 in, 2 out]
              }
            }
            n67 = local write "Set Centriod Target"(FALSE ("Set Centriod Target")) -> ()
          }
          event "stop": Value Change {
            # "Exit Button Value Change (pressed) Event\n(this executes Macro: Exit to terminate the VI)"
            n68 = event-data() -> ()  [unwired: 1 in, 6 out]
            n69 = Release Queue(queue=w150) -> (error out=w149:errorcluster)  [unwired: 2 in, 2 out]
            n70 = call <vilib>:"Clear Errors.vi"("error in (no error)"=w149) -> ()  [unwired: 6 in, 1 out]
            n71 = call <vilib>:"Add State(s) to Queue__jki_lib_state_machine.vi"("State(s) in Front (\"\")"="Macro: Exit", "State(s) in (\"\")"=w155) -> ("States Out"=w154:string)  [unwired: 13 in]
          }
          event Panel Close? {
            # "Discard the event because we'll close the front panel ourselves in Macro: Exit"
            # "Close Panel button (pressed) Event\n(this executes Macro: Exit to terminate the VI)"
            n72 = event-data() -> ()  [unwired: 1 in, 1 out]
            n73 = call <vilib>:"Add State(s) to Queue__jki_lib_state_machine.vi"("State(s) in Front (\"\")"="Macro: Exit", "State(s) in (\"\")"=w161) -> ("States Out"=w160:string)  [unwired: 13 in]
            n74 = event-data("Discard?"=TRUE) -> ()  [unwired: 1 in, 1 out]
          }
        }
      }
      frame "---------- Core ----------" {
        # "Do not put any code in this frame.\n(it is a separator no-op)"
        n75 = call <vilib>:"Add State(s) to Queue__jki_lib_state_machine.vi"("State(s) in (\"\")"=w165) -> ("States Out"=w164:string)  [unwired: 14 in]
      }
      frame Default {
        w175 = 42 items=["No error", "Argument error", "Memory is full", "Out of zone", "End of file", "File already open", "Generic file I/O error", "File not found", "File permission error", "Disk is full", "Duplicate path", "Too many files open", "System feature not enabled", "Resource file not found", "Cannot add resource", "Resource not found", "Image not found", "Image memory error", "Pen does not exist", "Config type invalid", "Config token not found", "Config parse error", "Config memory error", "Bad external code format", "Bad external code offset", "External code not present", "Null window", "Destroy window error", "Null menu", "Print aborted", "Bad print record", "Print driver error", "Windows error during printing", "Memory error during printing", "Print dialog error", "Generic print error", "Invalid device refnum", "Device not found", "Device parameter error", "Device unit error", "Cannot open device", "Device call aborted", "Generic error", "Cancelled by user", "Object ID too low", "Object ID too high", "Object not in heap", "Unknown heap", "Unknown object (invalid DefProc)", "Unknown object (DefProc not in table)", "Message out of range", "Invalid (null) method", "Unknown message", "Manager call not supported", "Bad address", "Network operation in progress", "Network operation timed out", "Connection is busy", "Network attribute not supported", "Network error", "Address in use", "System out of memory", "Connection aborted", "Connection refused", "Not connected", "Already connected", "Connection closed", "Initialization error (interapplication manager)", "Bad occurrence", "Wait on unbound occurrence handler", "Occurrence queue overflow", "Datalog type conflict", "Unused", "Unrecognized type (interapplication manager)", "Memory corrupt", "Failed to make temporary DLL", "Old CIN version", "Drag socket not found", "Failed to load drop-object", "Failed to register OLE object", "Failed to release OLE object", "Format specifier type mismatch", "Unknown format specifier", "Too few format specifiers", "Too many format specifiers", "Scan failed", "Newer CIN version", "Error converting to variant", "Runtime menu error", "Password tampered", "Variant attribute not found", "Incompatible variant data type", "Event data is not available", "Event Store is not present", "Occurrence is not found", "Event Queue is not created", "Event info is not available", "Refnum passed is NULL", "Error retrieving Class GUID", "Error retrieving CoClass GUID", "Error retrieving TypeLib GUID.", "Bad built application magic bytes.", "Specific driver is different from the specific driver associated with the Logical Name.", "There is no session opened to the class driver.", "Max Error", "MAX - Error with config objects", "MAX - Error loading configuration", "MAX - Group not supported"]
        # "Current State"
        # "Do not delete, rename, or modify this frame.\n(this is used to capture unhandled states and typos)"
        # "Handle mistyped state name (developer tool)"
        n76 = Format Into String(format string="Software Exception: Unhandled State \"%s\"." ("message"), error in=w171, w166) -> (resulting string=w174:string, error out=w173:errorcluster)  [unwired: 1 in]
        n77 = call <vilib>:"Error Cluster From Error Code.vi"("show call chain? (False)"=TRUE, "error in (no error)"=w173, "error message (\"\")"=w174, "error code (0)"=w175) -> ("error out"=w172:errorcluster)  [unwired: 5 in]
        n78 = call <vilib>:"Add State(s) to Queue__jki_lib_state_machine.vi"("State(s) in (\"\")"=w170) -> ("States Out"=w169:string)  [unwired: 14 in]
      }
      frame "Initialize Core Data" {
        # "Do not delete, rename, or modify this frame.\n(this is used to determine panel behavior on exit)"
        # "originally closed?"
        # "exe?"
        # "If panel starts closed or is an EXE, then close it when we exit"
        n79 = property class="VI"() -> ("Front Panel.Open"=w184:bool)  [unwired: 2 in, 2 out]
        n80 = property class="App"() -> ("App.Kind"=w183:T13)  [unwired: 2 in, 2 out]
        n81 = control-ref of="Current VI Reference"() -> (w177:refnum<vi>)
        n82 = Not(x=w184) -> (.not. x?=w181:bool)
        n83 = Equal?(x=w183, y=T13."Run Time System" ("Application:Kind")) -> (x = y?=w180:bool)
        n84 = Or(x=w181, y=w180) -> (x .or. y?=w178:bool)
        n85 = Bundle By Name(cluster=w179, "Core.Current VI Reference"=w177, "Core.Close Panel on Exit?"=w178) -> (w186:T17)
        n86 = call <vilib>:"Add State(s) to Queue__jki_lib_state_machine.vi"("State(s) in (\"\")"=w188) -> ("States Out"=w187:string)  [unwired: 14 in]
      }
      frame "Error Handler" {
        # "Unhandled Error -- Display it"
        # "Handle any errors here.\nYou can also output any states to clean-up after errors occur"
        # "Clear error"
        n87 = call <vilib>:"General Error Handler.vi"("error in (no error)"=w190) -> ()  [unwired: 10 in, 5 out]
        n88 = call <vilib>:"Add State(s) to Queue__jki_lib_state_machine.vi"("State(s) in Front (\"\")"="/* Post Error States", "State(s) in (\"\")"=w194) -> ("States Out"=w193:string)  [unwired: 13 in]
      }
      frame "Exit" {
        # "Do not put any code in this frame.\n(No errors that occur here will be handled.)"
        n89 = call <vilib>:"Add State(s) to Queue__jki_lib_state_machine.vi"("State(s) in (\"\")"=w199) -> ("States Out"=w198:string)  [unwired: 14 in]
      }
      frame "---------- Data ----------" {
        # "Do not put any code in this frame.\n(It is a separator no-op. You can make a copy of this frame to create a new Data frame)"
        n90 = call <vilib>:"Add State(s) to Queue__jki_lib_state_machine.vi"("State(s) in (\"\")"=w203) -> ("States Out"=w202:string)  [unwired: 14 in]
      }
      frame "Data: Initialize" {
        w204 = FALSE  # set centriod target
        w205 = T16 {"Stat Centriod X"=[], "Stat Centriod Y"=[], "TRA Position X"=[], "TRA PositionY"=[], "Time"=[]}  # Stats
        w208 = FALSE  # moving
        w207 = T5 {"Tolerance [%]"=0.0, "Stepsize"=0.0, "Invert Axis"=FALSE, "Invert Direction X"=FALSE, "Invert Direction Y"=FALSE, "enable feedback"=FALSE, "Set Centriod Target"=FALSE}  # move
        w209 = cluster{"X offset":dbl, "Y offset":dbl} {"X offset"=0.0, "Y offset"=0.0}  # offsets
        w210 = FALSE  # beam detected
        w206 = T3 {"Filter"=1, "Filter Para"={"X Size"=5, "Y Size"=5, "% Tolerance"=1}, "detection method"=4, "smal para"=[{"Measurement Parameter"=35, "Range Lower Value"=0.0, "Range Upper Value"=500.0, "Range"=TRUE, "Measurement Type"=FALSE}], "Remove small Objects"=TRUE, "Restrict to round Objects"=FALSE}  # beam detection para
        w211 = timestamp[] []  # Time
        w212 = dbl[] []  # Mean Centriod Y
        w213 = dbl[] []  # Mean Centriod X
        w214 = T6 [{"Area"=1104.0, "Number of Holes"=0.0, "Bounding Rect"={"Left"=378.0, "Top"=230.0, "Right"=422.0, "Bottom"=264.0}, "Center of Mass"={"X"=399.60235507246375, "Y"=246.169384057971}, "Orientation"=6.346766143267859, "Dimensions"={"Width"=44.0, "Height"=34.0}}]  # PArticle Report
        w215 = T8 []  # Best Rectangle
        w216 = dbl[] []  # Centriod Y
        w217 = dbl[] []  # Centriod X
        w218 = T19 {"Current VI Reference"=refnum, "Close Panel on Exit?"=FALSE}  # Core
        # "Initialize the shift-register data, here.\n(data names are defined by what you wire into the bundle function)"
        n91 = local write "beam detection para"(w206) -> ()
        n92 = Bundle("Core"=w218, "beam detection para"=w206, "Centriod X"=w217, "Centriod Y"=w216, "Best Rectangle"=w215, "PArticle Report"=w214, "Mean Centriod X"=w213, "Mean Centriod Y"=w212, "Time"=w211, "beam detected"=w210, "offsets"=w209, "move"=w207, "moving"=w208, "Stats"=w205, "set centriod target"=w204) -> (w220:T17)  [unwired: 1 in]
        n93 = call <vilib>:"Add State(s) to Queue__jki_lib_state_machine.vi"("State(s) in (\"\")"=w222) -> ("States Out"=w221:string)  [unwired: 14 in]
        n94 = local write "Move Properties"(w207) -> ()
      }
      frame "Data: Cleanup" {
        # "Cleanup any data and references, here.\n(this is called automatically, by the Macro: Exit)"
        n95 = Unbundle By Name(w224) -> ("Core.Current VI Reference"=w223:refnum<vi>)
        n96 = Close Reference(reference=w223, error in (no error)=w226) -> (error out=w225:errorcluster)
        n97 = call <vilib>:"Add State(s) to Queue__jki_lib_state_machine.vi"("State(s) in (\"\")"=w228) -> ("States Out"=w227:string)  [unwired: 14 in]
      }
      frame "---------- UI ----------" {
        # "Do not put any code in this frame.\n(It is a separator no-op. You can make a copy of this frame to create a new UI frame)"
        n98 = call <vilib>:"Add State(s) to Queue__jki_lib_state_machine.vi"("State(s) in (\"\")"=w232) -> ("States Out"=w231:string)  [unwired: 14 in]
      }
      frame "UI: Initialize" {
        # "Initialize the User Interface, here.\n(this is called automatically, by the Macro: Init)"
        n99 = call <vilib>:"Add State(s) to Queue__jki_lib_state_machine.vi"("State(s) in (\"\")"=w236) -> ("States Out"=w235:string)  [unwired: 14 in]
      }
      frame "UI: Cursor Set" {
        # "Argument"
        # "Set and Unset Cursor Busy.\n(Usage: \"UI: Cursor Set >> Busy|Idle\")"
        n100 = case shown="\"Idle\", Default" w237 {
          tunnel: w239 -> [w244 w246]
          tunnel: [w243 w245] -> w238
          frame "Idle", Default {
            n101 = call <vilib>:"Unset Busy.vi"("error in (no error)"=w244) -> ("error out"=w243:errorcluster)  [unwired: 10 in]
          }
          frame "Busy" {
            n102 = call <vilib>:"Set Busy.vi"("error in (no error)"=w246) -> ("error out"=w245:errorcluster)  [unwired: 9 in, 1 out]
          }
        }
        n103 = call <vilib>:"Add State(s) to Queue__jki_lib_state_machine.vi"("State(s) in (\"\")"=w242) -> ("States Out"=w241:string)  [unwired: 14 in]
      }
      frame "UI: Front Panel State" {
        # "Argument"
        # "Set Front Panel Open or Closed\n(Usage: \"UI: Front Panel State >> Open|Close\")"
        n104 = Unbundle By Name(w249) -> ("Core.Current VI Reference"=w248:refnum<vi>)
        n105 = case shown="\"Close\"" w247 {
          tunnel: w251 -> [w257 w270]
          tunnel: [w259 w271] -> w250
          tunnel: w248 -> [w258 w268]
          frame "Open", Default {
            n106 = property class="VI"(reference=w258, error in=w257) -> (reference out=w255:refnum<vi>, error out=w256:errorcluster, "Front Panel.Open"=w254:bool)
            n107 = case shown="False" w254 {
              tunnel: [w262 w265] -> w259
              tunnel: w256 -> [w261 w265]
              tunnel: w255 -> [w260 _]
              frame False {
                n108 = invoke class="VI" method="FP.Open"(reference=w260, error in=w261, "Activate"=TRUE, "State"=T14."Standard") -> (error out=w262:errorcluster)  [unwired: 1 in, 4 out]
              }
              frame True {
              }
            }
          }
          frame "Close" {
            n109 = property class="VI"(reference=w268, error in=w270) -> (reference out=w267:refnum<vi>, error out=w269:errorcluster, "Front Panel.Open"=w266:bool)
            n110 = case shown="True" w266 {
              tunnel: [w272 w275] -> w271
              tunnel: w269 -> [w272 w274]
              tunnel: w267 -> [_ w273]
              frame False {
              }
              frame True {
                n111 = invoke class="VI" method="FP.Close"(reference=w273, error in=w274) -> (error out=w275:errorcluster)  [unwired: 1 in, 2 out]
              }
            }
          }
        }
        n112 = call <vilib>:"Add State(s) to Queue__jki_lib_state_machine.vi"("State(s) in (\"\")"=w253) -> ("States Out"=w252:string)  [unwired: 14 in]
      }
      frame "---------- Macro ----------" {
        # "Do not put any code in this frame.\n(It is a separator no-op. You can make a copy of this frame to create a new Macro frame)"
        n113 = call <vilib>:"Add State(s) to Queue__jki_lib_state_machine.vi"("State(s) in (\"\")"=w279) -> ("States Out"=w278:string)  [unwired: 14 in]
      }
      frame "Macro: Initialize" {
        w280 = "Data: Initialize\nInitialize Core Data\nUI: Initialize\nUI: Front Panel State >> Open"  # Data: Initialize Initialize Core Data UI: Initialize UI: Front Panel State >> Open
        # "Initialization Macro\n(This is called once, when the VI starts)"
        n114 = call <vilib>:"Add State(s) to Queue__jki_lib_state_machine.vi"("State(s) in Front (\"\")"=w280, "State(s) in (\"\")"=w284) -> ("States Out"=w283:string)  [unwired: 13 in]
      }
      frame "Macro: Exit" {
        # "Exit Macro\n(This is called once, when the VI exits)"
        n115 = Unbundle By Name(w291) -> ("Core.Close Panel on Exit?"=w289:bool)
        n116 = Select(t="UI: Front Panel State >> Close", s=w289, f="") -> (s? t:f=w286:string)
        n117 = call <vilib>:"Add State(s) to Queue__jki_lib_state_machine.vi"("State(s) in (\"\")"=w286, "State(s) at Back (\"\")"="Data: Cleanup\nExit") -> ("States Out"=w290:string)  [unwired: 13 in]
        n118 = call <vilib>:"Add State(s) to Queue__jki_lib_state_machine.vi"("State(s) in Front (\"\")"=w290, "State(s) in (\"\")"=w294) -> ("States Out"=w293:string)  [unwired: 13 in]
      }
      frame "-------------Properties---------" {
        # "Template Separator\n(You can make a copy of, or modify, this frame)"
        n119 = call <vilib>:"Add State(s) to Queue__jki_lib_state_machine.vi"("State(s) in (\"\")"=w298) -> ("States Out"=w297:string)  [unwired: 14 in]
      }
      frame "Beam Detection" {
        # "Your code here.\n(You can make a copy of, or modify, this frame)"
        n120 = Bundle By Name(cluster=w300, "beam detection para"="beam detection para") -> (w299:T17)
        n121 = call <vilib>:"Add State(s) to Queue__jki_lib_state_machine.vi"("State(s) in (\"\")"=w304) -> ("States Out"=w303:string)  [unwired: 14 in]
      }
      frame "Move Properties" {
        n122 = Bundle By Name(cluster=w306, "move"="Move Properties") -> (w305:T17)
        n123 = call <vilib>:"Add State(s) to Queue__jki_lib_state_machine.vi"("State(s) in (\"\")"=w310) -> ("States Out"=w309:string)  [unwired: 14 in]
      }
      frame "Save Configuration" {
        n124 = Unbundle By Name(w321) -> ("beam detection para"=w319:T3, "move"=w318:T5)
        n125 = local read "img to avg"() -> (w320:i32)
        n126 = Bundle("img to avg"=w320, "beam detection para"=w319, "move"=w318) -> (w317:T7)  [unwired: 1 in]
        n127 = Open/Create/Replace File(error in=w313, operation (0:open)=T15."replace or create with confirmation") -> (refnum out=w322:refnum<file>, error out=w316:errorcluster)  [unwired: 4 in, 1 out]
        n128 = Write to Binary File(file (use dialog)=w322, data=w317, error in=w316) -> (refnum out=w314:refnum<file>, error out=w315:errorcluster)  [unwired: 3 in, 1 out]
        n129 = Close File(refnum=w314, error in=w315) -> (error out=w312:errorcluster)  [unwired: 1 out]
        n130 = local write "Save Config"(FALSE ("Save Button")) -> ()
        n131 = call <vilib>:"Add State(s) to Queue__jki_lib_state_machine.vi"("State(s) in (\"\")"=w325) -> ("States Out"=w324:string)  [unwired: 14 in]
      }
      frame "Save Stats" {
        n132 = Unbundle By Name(w333) -> ("Stats"=w326:T16)
        n133 = Open/Create/Replace File(error in=w329, operation (0:open)=T15."replace or create with confirmation") -> (refnum out=w334:refnum<file>, error out=w332:errorcluster)  [unwired: 4 in, 1 out]
        n134 = Write to Binary File(file (use dialog)=w334, data=w326, error in=w332) -> (refnum out=w330:refnum<file>, error out=w331:errorcluster)  [unwired: 3 in, 1 out]
        n135 = Close File(refnum=w330, error in=w331) -> (error out=w328:errorcluster)  [unwired: 1 out]
        n136 = call <vilib>:"Add State(s) to Queue__jki_lib_state_machine.vi"("State(s) in (\"\")"=w337) -> ("States Out"=w336:string)  [unwired: 14 in]
        n137 = local write "Save Stats"(FALSE ("Save Button")) -> ()
      }
      frame "Load Configuration" {
        # "Your code here.\n(You can make a copy of, or modify, this frame)"
        n138 = Open/Create/Replace File(error in=w342, operation (0:open)=T15."open") -> (refnum out=w350:refnum<file>, error out=w349:errorcluster)  [unwired: 4 in, 1 out]
        n139 = Read from Binary File(5:"save cluster", 8:w349, 11:w350) -> (0:w348:errorcluster, 2:w345:T7, 3:w347:refnum<file>)  [unwired: 3 in, 1 out]
        n140 = Close File(refnum=w347, error in=w348) -> (error out=w341:errorcluster)  [unwired: 1 out]
        n141 = Unbundle By Name(w345) -> ("beam detection para"=w340:T3, "move"=w339:T5)  [unwired: 1 out]
        n142 = Bundle By Name(cluster=w344, "beam detection para"=w340, "move"=w339) -> (w343:T17)
        n143 = local write "beam detection para"(w340) -> ()
        n144 = local write "Move Properties"(w339) -> ()
        n145 = call <vilib>:"Add State(s) to Queue__jki_lib_state_machine.vi"("State(s) in (\"\")"=w353) -> ("States Out"=w352:string)  [unwired: 14 in]
        n146 = local write "Load Config"(FALSE ("Load Button")) -> ()
      }
      frame "Reset History" {
        w357 = dbl[] [] ("Mean Centriod X")
        # "Your code here.\n(You can make a copy of, or modify, this frame)"
        n147 = local write "Reset History"(FALSE ("Reset History")) -> ()
        n148 = call <vilib>:"Add State(s) to Queue__jki_lib_state_machine.vi"("State(s) in (\"\")"=w360) -> ("States Out"=w359:string)  [unwired: 14 in]
        n149 = Bundle By Name(cluster=w356, "Mean Centriod X"=w357, "Mean Centriod Y"=w357) -> (w355:T17)
      }
      frame "---------- centriod analysis----------" {
        # "Template Separator\n(You can make a copy of, or modify, this frame)"
        n150 = call <vilib>:"Add State(s) to Queue__jki_lib_state_machine.vi"("State(s) in (\"\")"=w364) -> ("States Out"=w363:string)  [unwired: 14 in]
      }
      frame "detected" {
        w388 = dbl[] [] ("Array")
        n151 = Unbundle By Name(w371) -> ("Time"=w381:timestamp[], "Centriod X"=w376:dbl[], "Mean Centriod X"=w380:dbl[], "Centriod Y"=w375:dbl[], "Mean Centriod Y"=w379:dbl[], "Best Rectangle"=→"Best Rectangle":T8)
        n152 = local read "Target.X::1"() -> (w378:dbl)
        n153 = local read "Target.Y::1"() -> (w377:dbl)
        n154 = call <vilib>:"Std Deviation and Variance.vi"("X"=w376) -> ("mean"=w382:dbl)  [unwired: 1 in, 2 out]
        "mean X" <- w382
        n155 = call <vilib>:"Std Deviation and Variance.vi"("X"=w375) -> ("mean"=w383:dbl)  [unwired: 1 in, 2 out]
        "mean Y" <- w383
        n156 = Subtract(x=w378, y=w382) -> (x-y=w369:dbl)
        "X offset" <- w369
        n157 = Subtract(x=w377, y=w383) -> (x-y=w368:dbl)
        "Y offset" <- w368
        n158 = Get Date/Time In Seconds() -> (seconds since 1Jan1904=w384:timestamp)
        n159 = Build Array (concatenate)(w380, w369) -> (w373:dbl[])
        n160 = Build Array (concatenate)(w379, w368) -> (w372:dbl[])
        n161 = Build Array (concatenate)(w381, w384) -> (w374:timestamp[])
        n162 = Bundle(w369, w368) -> (w367:cluster{dbl, dbl})  [unwired: 1 in]
        n163 = Bundle(w374, w373) -> (w385:cluster{timestamp[], dbl[]})  [unwired: 1 in]
        n164 = Bundle(w374, w372) -> (w386:cluster{timestamp[], dbl[]})  [unwired: 1 in]
        n165 = call <vilib>:"Add State(s) to Queue__jki_lib_state_machine.vi"("State(s) in (\"\")"=w391, "State(s) at Back (\"\")"="check move") -> ("States Out"=w390:string)  [unwired: 13 in]
        n166 = Build Array(w385, w386) -> (→"XY Graph":cluster{timestamp[], dbl[]}[])
        n167 = Bundle By Name(cluster=w371, "Time"=w374, "Mean Centriod X"=w373, "Mean Centriod Y"=w372, "Centriod X"=w388, "Centriod Y"=w388, "offsets"=w367) -> (w370:T17)
      }
      frame "check move" {
        n168 = Unbundle By Name(w398) -> ("Best Rectangle"=w416:T8, "offsets.X offset"=w415:dbl, "offsets.Y offset"=w414:dbl)
        n169 = Absolute Value(x=w415) -> (abs(x)=w411:dbl)
        n170 = Absolute Value(x=w414) -> (abs(x)=w408:dbl)
        n171 = Unbundle By Name(w398) -> ("move.Tolerance [%]"=w413:dbl)
        n172 = call "Beam Size.vi"("Best Rectangle"=w416) -> ("Y Size"=w394:dbl, "X Size"=w395:dbl)  [unwired: 9 in]
        "X Size" <- w395
        "Y Size" <- w394
        n173 = Divide(x=w413, y=100.0) -> (x/y=w409:dbl)
        n174 = Multiply(x=w409, y=w395) -> (x*y=w410:dbl)
        n175 = Multiply(x=w409, y=w394) -> (x*y=w407:dbl)
        n176 = Max & Min(x=w395, y=w394) -> (max(x,y)=w393:dbl)  [unwired: 1 out]
        n177 = Divide(x=w393, y=2.0) -> ()  [unwired: 1 out]
        n178 = Greater Or Equal?(x=w411, y=w410) -> (x >= y?=w401:bool)
        n179 = Greater Or Equal?(x=w408, y=w407) -> (x >= y?=w400:bool)
        n180 = case shown="True" w400 {
          tunnel: w396 -> [w423 w426]
          tunnel: [w423 w424] -> w406
          frame False {
          }
          frame True {
            n181 = call <vilib>:"Add State(s) to Queue__jki_lib_state_machine.vi"("State(s) in (\"\")"=w426, "State(s) at Back (\"\")"="Move Y" ("State(s) at Back (\"\")")) -> ("States Out"=w424:string)  [unwired: 13 in]
          }
        }
        n182 = case shown="True" w401 {
          tunnel: w396 -> [w427 w430]
          tunnel: [w427 w428] -> w405
          frame False {
          }
          frame True {
            n183 = call <vilib>:"Add State(s) to Queue__jki_lib_state_machine.vi"("State(s) in (\"\")"=w430, "State(s) at Back (\"\")"="Move X" ("State(s) at Back (\"\")")) -> ("States Out"=w428:string)  [unwired: 13 in]
          }
        }
        n184 = Or(x=w401, y=w400) -> (x .or. y?=w399:bool)
        n185 = Unbundle By Name(w398) -> ("move.enable feedback"=w397:bool)
        n186 = local write "move required"(w399) -> ()
        n187 = Bundle By Name(cluster=w398, "Best Rectangle"=T8 []) -> (w402:T17)
        n188 = case shown="True" w397 {
          tunnel: w406 -> [_ w422]
          tunnel: w405 -> [_ w421]
          tunnel: [w418 w420] -> w404
          tunnel: w396 -> [w418 _]
          frame False {
          }
          frame True {
            n189 = call <vilib>:"Add State(s) to Queue__jki_lib_state_machine.vi"("State(s) in Front (\"\")"="Wait2" ("State(s) in Front (\"\")"), "State(s) in (\"\")"=w421, "State(s) at Back (\"\")"=w422) -> ("States Out"=w420:string)  [unwired: 12 in]
          }
        }
      }
      frame "-----------Motor Move---------" {
        # "Your code here.\n(You can make a copy of, or modify, this frame)"
        n190 = call <vilib>:"Add State(s) to Queue__jki_lib_state_machine.vi"("State(s) in (\"\")"=w434) -> ("States Out"=w433:string)  [unwired: 14 in]
      }
      frame "Move X" {
        w438 = TRUE ("moving")
        n191 = Unbundle By Name(w437) -> ("move.Invert Direction X"=w444:bool, "move.Invert Axis"=w442:bool, "move.Stepsize"=w443:dbl, "offsets.X offset"=w436:dbl)
        "move.Stepsize" <- w443
        n192 = Greater Than 0?(x=w436) -> (x > 0?=w435:bool)
        n193 = Unbundle By Name(w437) -> ("move.Invert Axis"=w441:bool)
        n194 = case shown="False" w435 {
          tunnel: w444 -> [w453 w469]
          tunnel: w443 -> [w451 w467]
          tunnel: w442 -> [w450 w466]
          tunnel: w441 -> [w449 w465]
          frame True {
            n195 = case shown="True" w450 {
              tunnel: [w462 w463] -> w452
              frame False {
                n196 = local read "Position.Axis 1::2"() -> (w462:dbl)
              }
              frame True {
                n197 = local read "Position.Axis 2::2"() -> (w463:dbl)
              }
            }
            n198 = case shown="True" w453 {
              tunnel: w452 -> [w458 w461]
              tunnel: w451 -> [w457 w460]
              tunnel: [w456 w459] -> w448
              frame False {
                n199 = Add(x=w458, y=w457) -> (x+y=w456:dbl)
              }
              frame True {
                n200 = Subtract(x=w461, y=w460) -> (x-y=w459:dbl)
              }
            }
            n201 = case shown="True" w449 {
              tunnel: w448 -> [w454 w455]
              frame False {
                n202 = property on="Position.Axis 1::2" class="DigNum (strict)"("Val(Sgnl)"=w454) -> ()  [unwired: 2 in, 2 out]
              }
              frame True {
                n203 = property on="Position.Axis 2::2" class="DigNum (strict)"("Val(Sgnl)"=w455) -> ()  [unwired: 2 in, 2 out]
              }
            }
          }
          frame False {
            n204 = case shown="True" w466 {
              tunnel: [w478 w479] -> w468
              frame False {
                n205 = local read "Position.Axis 1::2"() -> (w478:dbl)
              }
              frame True {
                n206 = local read "Position.Axis 2::2"() -> (w479:dbl)
              }
            }
            n207 = case shown="False" w469 {
              tunnel: w468 -> [w474 w477]
              tunnel: w467 -> [w473 w476]
              tunnel: [w472 w475] -> w464
              frame False {
                n208 = Subtract(x=w474, y=w473) -> (x-y=w472:dbl)
              }
              frame True {
                n209 = Add(x=w477, y=w476) -> (x+y=w475:dbl)
              }
            }
            n210 = case shown="True" w465 {
              tunnel: w464 -> [w470 w471]
              frame False {
                n211 = property on="Position.Axis 1::2" class="DigNum (strict)"("Val(Sgnl)"=w470) -> ()  [unwired: 2 in, 2 out]
              }
              frame True {
                n212 = property on="Position.Axis 2::2" class="DigNum (strict)"("Val(Sgnl)"=w471) -> ()  [unwired: 2 in, 2 out]
              }
            }
          }
        }
        n213 = call <vilib>:"Add State(s) to Queue__jki_lib_state_machine.vi"("State(s) in Front (\"\")"="Wait", "State(s) in (\"\")"=w447) -> ("States Out"=w446:string)  [unwired: 13 in]
        n214 = Bundle By Name(cluster=w437, "moving"=w438) -> (w439:T17)
        n215 = local write "moving"(w438) -> ()
      }
      frame "Move Y" {
        w484 = TRUE ("moving")
        n216 = Unbundle By Name(w483) -> ("move.Invert Direction Y"=w489:bool, "move.Invert Axis"=w487:bool, "move.Stepsize"=w488:dbl, "offsets.Y offset"=w481:dbl)
        "move.Stepsize 2" <- w488
        n217 = Greater Than 0?(x=w481) -> (x > 0?=w480:bool)
        n218 = Unbundle By Name(w483) -> ("move.Invert Axis"=w486:bool)
        n219 = case shown="True" w480 {
          tunnel: w489 -> [w498 w514]
          tunnel: w488 -> [w496 w512]
          tunnel: w487 -> [w495 w511]
          tunnel: w486 -> [w494 w510]
          frame True {
            n220 = case shown="False" w495 {
              tunnel: [w507 w508] -> w497
              frame False {
                n221 = local read "Position.Axis 2::2"() -> (w507:dbl)
              }
              frame True {
                n222 = local read "Position.Axis 1::2"() -> (w508:dbl)
              }
            }
            n223 = case shown="True" w498 {
              tunnel: w497 -> [w503 w506]
              tunnel: w496 -> [w502 w505]
              tunnel: [w501 w504] -> w493
              frame False {
                n224 = Add(x=w503, y=w502) -> (x+y=w501:dbl)
              }
              frame True {
                n225 = Subtract(x=w506, y=w505) -> (x-y=w504:dbl)
              }
            }
            n226 = case shown="True" w494 {
              tunnel: w493 -> [w499 w500]
              frame False {
                n227 = property on="Position.Axis 2::2" class="DigNum (strict)"("Val(Sgnl)"=w499) -> ()  [unwired: 2 in, 2 out]
              }
              frame True {
                n228 = property on="Position.Axis 1::2" class="DigNum (strict)"("Val(Sgnl)"=w500) -> ()  [unwired: 2 in, 2 out]
              }
            }
          }
          frame False {
            n229 = case shown="True" w511 {
              tunnel: [w523 w524] -> w513
              frame False {
                n230 = local read "Position.Axis 2::2"() -> (w523:dbl)
              }
              frame True {
                n231 = local read "Position.Axis 1::2"() -> (w524:dbl)
              }
            }
            n232 = case shown="True" w514 {
              tunnel: w513 -> [w519 w522]
              tunnel: w512 -> [w518 w521]
              tunnel: [w517 w520] -> w509
              frame False {
                n233 = Subtract(x=w519, y=w518) -> (x-y=w517:dbl)
              }
              frame True {
                n234 = Add(x=w522, y=w521) -> (x+y=w520:dbl)
              }
            }
            n235 = case shown="True" w510 {
              tunnel: w509 -> [w515 w516]
              frame False {
                n236 = property on="Position.Axis 2::2" class="DigNum (strict)"("Val(Sgnl)"=w515) -> ()  [unwired: 2 in, 2 out]
              }
              frame True {
                n237 = property on="Position.Axis 1::2" class="DigNum (strict)"("Val(Sgnl)"=w516) -> ()  [unwired: 2 in, 2 out]
              }
            }
          }
        }
        n238 = call <vilib>:"Add State(s) to Queue__jki_lib_state_machine.vi"("State(s) in Front (\"\")"="Wait", "State(s) in (\"\")"=w492) -> ("States Out"=w491:string)  [unwired: 13 in]
        n239 = Bundle By Name(cluster=w483, "moving"=w484) -> (w482:T17)
        n240 = local write "moving"(w484) -> ()
      }
      frame "Wait" {
        w528 = TRUE ("moving")
        # "Wait as long as the motor is moving"
        n241 = while {
          tunnel: w529 -> [w542]
          tunnel: [w542] -> w526
          stop <- w533 stop-if-true
          w538 = StatusTRA_TypDef."DISABLE" ("y")
          n242 = local read "Status.Axis 3::2"() -> (w543:T1)
          n243 = local read "Status.Axis 4::2"() -> (w541:T1)
          n244 = local read "Status.Axis 1::2"() -> (w540:T1)
          n245 = local read "Status.Axis 2::2"() -> (w539:T1)
          n246 = Equal?(x=w543, y=w538) -> (x = y?=w537:bool)
          n247 = Equal?(x=w541, y=w538) -> (x = y?=w536:bool)
          n248 = Equal?(x=w538, y=w540) -> (x = y?=w535:bool)
          n249 = Equal?(x=w538, y=w539) -> (x = y?=w534:bool)
          n250 = Compound Arithmetic op=AND(w537, w536, w535, w534) -> (w533:bool)
        }
        n251 = call <vilib>:"Add State(s) to Queue__jki_lib_state_machine.vi"("State(s) in (\"\")"=w532, "State(s) at Back (\"\")"="Stats" ("State(s) at Back (\"\")")) -> ("States Out"=w531:string)  [unwired: 13 in]
        n252 = Bundle By Name(cluster=w526, "moving"=w528) -> (w527:T17)
        n253 = local write "moving"(w528) -> ()
      }
      frame "Wait2" {
        # "Wait as long as the motor is moving"
        n254 = while {
          tunnel: w545 -> [w558]
          tunnel: [w558] -> w544
          stop <- w549 stop-if-true
          w554 = StatusTRA_TypDef."DISABLE" ("y")
          n255 = local read "Status.Axis 3::2"() -> (w559:T1)
          n256 = local read "Status.Axis 4::2"() -> (w557:T1)
          n257 = local read "Status.Axis 1::2"() -> (w556:T1)
          n258 = local read "Status.Axis 2::2"() -> (w555:T1)
          n259 = Equal?(x=w559, y=w554) -> (x = y?=w553:bool)
          n260 = Equal?(x=w557, y=w554) -> (x = y?=w552:bool)
          n261 = Equal?(x=w554, y=w556) -> (x = y?=w551:bool)
          n262 = Equal?(x=w554, y=w555) -> (x = y?=w550:bool)
          n263 = Compound Arithmetic op=AND(w553, w552, w551, w550) -> (w549:bool)
        }
        n264 = call <vilib>:"Add State(s) to Queue__jki_lib_state_machine.vi"("State(s) in (\"\")"=w548) -> ("States Out"=w547:string)  [unwired: 14 in]
      }
      frame "Stats" {
        # "Your code here.\n(You can make a copy of, or modify, this frame)"
        n265 = Unbundle By Name(w582) -> ("Stats.TRA Position X"=w587:dbl[], "Stats.TRA PositionY"=w586:dbl[], "Stats.Stat Centriod X"=w579:dbl[], "Mean Centriod Y"=w578:dbl[], "Stats.Time"=w574:timestamp[])
        n266 = local read "Position.Axis 2::2"() -> (w585:dbl)
        n267 = local read "Position.Axis 1::2"() -> (w584:dbl)
        n268 = local read "Y offset"() -> (w576:dbl)
        n269 = local read "X offset"() -> (w577:dbl)
        n270 = Get Date/Time In Seconds() -> (seconds since 1Jan1904=w573:timestamp)
        n271 = Wait (ms)(milliseconds to wait="wait") -> ()  [unwired: 1 out]
        n272 = Build Array (concatenate)(w586, w585) -> (w581:dbl[])
        n273 = Build Array (concatenate)(w579, w577) -> (w580:dbl[])
        n274 = Build Array (concatenate)(w578, w576) -> (w575:dbl[])
        n275 = Build Array (concatenate)(w574, w573) -> (w572:timestamp[])
        n276 = Build Array (concatenate)(w587, w584) -> (w583:dbl[])
        n277 = Bundle By Name(cluster=w582, "Stats.TRA Position X"=w583, "Stats.TRA PositionY"=w581, "Stats.Stat Centriod X"=w580, "Stats.Stat Centriod Y"=w575, "Stats.Time"=w572) -> (w571:T17)
        n278 = Unbundle By Name(w571) -> ("Stats.Time"=w567:timestamp[], "Stats.Stat Centriod X"=w570:dbl[], "Stats.Stat Centriod Y"=w569:dbl[], "Stats.TRA Position X"=w568:dbl[], "Stats.TRA PositionY"=w566:dbl[])
        n279 = call <vilib>:"Add State(s) to Queue__jki_lib_state_machine.vi"("State(s) in (\"\")"=w590) -> ("States Out"=w589:string)  [unwired: 14 in]
        n280 = Bundle("Time"=w567, "Stat Centriod X"=w570) -> (w565:T20)  [unwired: 1 in]
        n281 = Bundle("Time"=w567, "Stat Centriod Y"=w569) -> (w564:T21)  [unwired: 1 in]
        n282 = Bundle("Time"=w567, "TRA Position X"=w568) -> (w563:T22)  [unwired: 1 in]
        n283 = Bundle("Time"=w567, "TRA PositionY"=w566) -> (w562:T23)  [unwired: 1 in]
        n284 = Build Array(w565, w564, w563, w562) -> (→"Stats":T24)
      }
      frame "New Category: 2" {
        # "Your code here.\n(You can make a copy of, or modify, this frame)"
        n285 = call <vilib>:"Add State(s) to Queue__jki_lib_state_machine.vi"("State(s) in (\"\")"=w594) -> ("States Out"=w593:string)  [unwired: 14 in]
      }
    }
  }
  n286 = call <vilib>:"Clear Errors.vi"("error in (no error)"=w18) -> ("error out"=w16:errorcluster)  [unwired: 6 in]
  n287 = call "IMAQ Dispose"("error in (no error)"=w16) -> ("error out"=w15:errorcluster)  [unwired: 5 in]
  n288 = call "IMAQ Dispose"("Image"=w11, "error in (no error)"=w15) -> ("error out"=→"error IO 2":errorcluster)  [unwired: 4 in]
